vi "Dashboard Main.vi"() -> ()   [LabVIEW 2015]
uses:
  <vilib>/Rock Robotics/Network Tables/NT Read Boolean.vi
  <vilib>/Utility/config.llb/Write Key (String).vi
  <vilib>/Utility/config.llb/Write Key (I32).vi
  <vilib>/event_ctls.llb/eventvkey.ctl
  <vilib>/Utility/config.llb/NI_LVConfig.lvlib
  <vilib>/Rock Robotics/WPI/Dashboard/WPI_DashboardLogging Global.vi
  <vilib>/vision/NI_Vision_Development_Module.lvlib
panel:
  in  "LED Robot Mode":T1(ring)
  out "leds 1":string="RGB LED Control                                                                 "
  in  "LEDs OFF":bool caption="Tare PDP Currents:\nSets current currents to zero,\nlike homing a scale."
  in  "Opening Ceremonies Mode":bool caption="Tare PDP Currents:\nSets current currents to zero,\nlike homing a scale."
  out "leds 2":string="LED Mode Override                                                             "
  in  "Override LED Mode":bool caption="Tare PDP Currents:\nSets current currents to zero,\nlike homing a scale."
  out "leds 3":string="Opening ceremonies mode takes precedence over the mode set using override LED mode."
  out "Chart 2":cluster{"Numeric":dbl, "Numeric":dbl}(graph)
  in  "Notifications":bool
  in  "NotificationCluster":cluster{"Notification Log":i32[]}
  out "notification":string
  out "Robot Mode":T2(ring)
  out "Process?":bool
  in  "Listbox":i32(listbox)
  out "Progress":T3 {"Test Progress" scale=0.0..100.0}
  in  "Motor":cluster{"Value":dbl, "Enable":bool} {"Value" scale=-1.0..1.0 scale format="%#_3g"}
  in  "Test Slider":dbl(slide) scale=0.0..100.0 scale format="%#_3g"
  in  "On/Off":bool caption="Solenoid"
  in  "Test Name":u16(ring) items=["Select the test to run..."]
  in  "Rev/Fwd":cluster{"Forward":bool, "Reverse":bool}
  in  "Test Ring":u16(ring) items=["Monochrome", "Color"]
  in  "Test Tree":string(tree)
  in  "DB/String 9":string
  in  "DB/String 8":string
  in  "DB/String 7":string
  in  "DB/String 6":string
  in  "DB/String 5":string
  in  "DB/String 4":string
  in  "DB/String 3":string
  in  "DB/String 2":string
  in  "DB/String 1":string
  in  "DB/String 0":string
  in  "DB/Slider 0":dbl(slide) scale=0.0..5.0
  in  "DB/Slider 1":dbl(slide) scale=0.0..5.0
  in  "DB/Slider 2":dbl(slide) scale=0.0..5.0
  in  "DB/Slider 3":dbl(slide) scale=0.0..5.0
  out "DB/LED 3":bool
  out "DB/LED 2":bool
  out "DB/LED 1":bool
  out "DB/LED 0":bool
  in  "DB/Button 3":bool
  in  "DB/Button 2":bool
  in  "DB/Button 1":bool
  in  "DB/Button 0":bool caption="New Name"
  in  "TCP":refnum<k5>
  in  "Rec Mode":enum32{"Stop", "Record", "Playback"}(radio)
  out "Camera IP":string
  in  "Dashboard Tab":T4(tab)
  out "Shooter Camera Active":bool
  out "Intake Camera Active":bool
  out "Camera In Targeting Mode":bool
  out "Intake Ball Sensor":bool
  in  "Camera Selector":bool=TRUE
  out "Robot Mode 2":T2(ring)=enum."Disconnected"
  in  "Camera Settings":T5={"Frame Rate"=30, "Compression"=30, "Size"=1} {"Size" items=["640x480", "320x240", "160x120"]; "Frame Rate" scale=1.0..30.0}
  out "Image Message":string="Timeout in Camera Communications"
  out "Camera Image":T6(plugin-control)
  in  "DB Camera Config":bool
  out "fps":dbl format="%#.1g"
  out "Mbps 2":bool
  out "FMS Connection":bool
  out "Dashboard Connection":bool
  out "Robot Connection":bool
  in  "Vision":u16(ring)=2 items=["Camera Off", "USB Camera SW", "USB Camera HW", "IP Camera"]
  out "Mbps":i32 format="%.0f mb/s"
  out "Arm Actuator \nLimit Switches":cluster{"Back":bool, "Forward":bool}
  out "Chart":cluster{"Distance":dbl, "Distance":dbl}(graph)
  out "Gyro":dbl(knob) scale=0.0..360.0 scale format="%#_g°"
  out "Angle":dbl format="%#_g°"
  out "Angular Rate (°/s)":dbl
  in  "Right":bool
  in  "Left":bool
  out "Left Drive":cluster{"Distance":dbl, "Rate":dbl} {"Distance" format="%#_g in"}
  out "MotorSliders L":cluster{"MotorSlide4 2":dbl} {"MotorSlide4 2" scale=0.0..14.0 scale format="%#_2e"}
  out "MotorChart L":cluster{"Battery V":dbl}(graph)
  out "Right Drive":cluster{"Distance":dbl, "Rate":dbl} {"Distance" format="%#_g in"}
  out "Robot IP":string
  out "Camera IP":string
  out "Shooter Rate":dbl format="%#_g rpm"
  out "Arm Actuator Rate":dbl
  out "Arm Actuator Distance":dbl
  out "Targets":T6(plugin-control)
  out "Image":T6(plugin-control)
  in  "Hue Range":cluster{"Lower value":i32, "Upper value":i32}={"Lower value"=80, "Upper value"=120}
  in  "Sat Range":cluster{"Lower value":i32, "Upper value":i32}={"Lower value"=52, "Upper value"=255}
  in  "Luma Range":cluster{"Lower value":i32, "Upper value":i32}={"Lower value"=40, "Upper value"=255}
  out "safety info":string="See Error Log page for more information."
  out "Drive Train":T7
  out "Arm Actuator":T8
  out "Ramp Belts":T9
  out "Shooter":T10
  in  "Error Log":i32(listbox)=-1
  out "CPU Utilization":T11 {"CPU % ISR" format="%#_g%"; "CPU % Time Crit" format="%#_g%"; "CPU % Timed Str" format="%#_g%"; "CPU % High" format="%#_g%"; "CPU % Above" format="%#_g%"; "CPU % Normal" format="%#_g%"; "CPU % Low" format="%#_g%"}
  out "RAM Usage":u32(slide) max=0 scale=-1.0..242810880.0
  out "CPU %":sgl(slide) scale=0.0..100.0
  out "CAN":T12 {"% Bus Utilization" format="%#_g%"}
  out "CAN BUS %":sgl(slide) scale=0.0..100.0
  out "Storage":T13
  out "Current":dbl format="%#_gA"
  out "Temperature":dbl format="%#_g°F"
  out "roboRIO":T14 {"roboRIO V&I"."roboRIO input voltage" format="%#_gV"; "roboRIO V&I"."roboRIO input current" format="%#_gA"}
  out "Rail Voltages":T15 {"6 volt rail"."6 volt rail voltage" format="%#_gV"; "6 volt rail"."6 volt rail current" format="%#_gA"; "5 volt rail"."5 volt rail voltage" format="%#_gV"; "5 volt rail"."5 volt rail current" format="%#_gA"; "3.3 volt rail"."3.3 volt rail voltage" format="%#_gV"; "3.3 volt rail"."3.3 volt rail current" format="%#_gA"}
  out "All Currents (A)":dbl[](array[numeric])
  out "Voltage":dbl format="%#_gV"
  out "PDP Energy":cluster{"Energy":dbl, "Power":dbl} {"Energy" format="%#_gJ"; "Power" format="%#_gW"}
  out "Control Bits":T16
  out "Status Bits":T17
  out "Team Station":u8(ring) items=["Red 1", "Red 2", "Red 3", "Blue 1", "Blue 2", "Blue 3"]
  out "Countdown":sgl
  out "Match Replay":u8
  out "Match Number":u16
  out "Match Type":u8
  out "Event Name":string
  out "Code Trace":T18
  out "Code?":enum16{"unknown", "noCode", "code"}(ring)
  out "Controller Type":enum16{"unknown", "cRIO", "roboRio"}(ring)
  out "Tree":string(tree)
  in  "refresh":bool
  out "Keys":string[](array[string])
  in  "Values":string[](array[string])
  in  "update":bool
  in  "Enable Compressor":bool
  in  "What should the robot do?":T19(ring)
  in  "What defense is in front of the robot?":T20(ring)
  in  "Clear Log":bool caption="Clear Log: This clears the notification\nlog."
  in  "Bottom Right":bool caption="Bottom Right: Moves the notification\nbar to the  bottom right of the screen."
  in  "Bottom Left":bool caption="Bottom Left: Moves the notification\nbar to the bottom left of the screen."
  in  "Top Right":bool caption="Top Right: Moves the notification\nbar to the top right of the screen."
  in  "Top Left":bool caption="Top Left: Moves the notification\nbar to the top left of the screen."
  out "Notifications":bool
  in  "Enable Notifications":bool=TRUE caption="Enable Notifications: Enable the\ndisplaying of important power\nwarnings in a notification pop-up."
  out "hover hint":string="hover over controls for help"
  out "About Selected Auto Mode":string
  in  "Reset Error Log":bool caption="Reset Error Log:\nThis clears all the entries in the error \nlog on the error log tab."
  in  "Clear PDP Sticky Faults":bool caption="Clear PDP Sticky Faults:\nThis resets the faults on the PDP and \nthe associated LEDs. These faults do \nnot clear with a robot reboot."
  in  "Reset PDP Energy":bool caption="Reset PDP Energy:\nResets the PDP energy statistics,\nspecifically the energy (J) and the\npower (W)."
  in  "Dismiss Notification":bool caption="Dismiss Notification: Clears the\ncurrent notification."
  in  "Which defense position is the robot in front of?":enum16{"1", "2", "3", "4", "5", "Spy Box"}(ring)=enum."2"
  out "Dashboard Revision":string
  out "What's connected?":string
  in  "Channel":T21(ring)
  out "Code Revision":string
  out "Time":string
  out "Boolean":bool
  # "1124"
  # "Connections & Robot Status"
  # "Robot Name Goes Here     换"
  # "Don't forget to configure autonomous!"
  # "««       Build Season Alpha Build         »»"
  # "Intake Camera"
  # "Shooter Camera"
  # "General"
  # "Arm Actuator"
  # "Shooter Wheels"
  # "Battery"
  # "Battery"
  # "Default\nValues"
  # "80\n\n\n120"
  # "52\n\n\n255"
  # "40\n\n\n255"
  # "Robot Metrics"
  # "See the below driver station for\ngraphs of CPU%"
  # "PDP Data"
  # "General"
  # "Event & Match Info"
  # "This controls the roboRIO's local config file and \npersists after reboots. \n\nThis data is roboRIO\nspecific and only affects the currently connected\nroboRIO. \n\nOnly edit these if you know what you are doing.\nPlease."
  # "Power Commands"
  # "Notifications"
  # "Power Distribution Panel"
  # "Only do this when\nthe compressor\nis connected!"
  # "Autonomous Configuration"
  # "Error Log Controls"
  # "Screen Location"
  # "Help"
  # "Power Distribution Panel Channels"
  # "ÜberBots Team 1124"
  # "CAN Line for Talon SRX in Parentheses if Applicable"
  # "ÜberDashboard 2015"
  # "Power Distribution Panel"
  # "CH 0"
  # "CH 3"
  # "CH 2"
  # "CH 1"
  # "CH 6"
  # "CH 7"
  # "CH 5"
  # "CH 4"
  # "CH 12"
  # "CH 13"
  # "CH 14"
  # "CH 15"
  # "CH 8"
  # "CH 9"
  # "CH 10"
  # "CH 11"
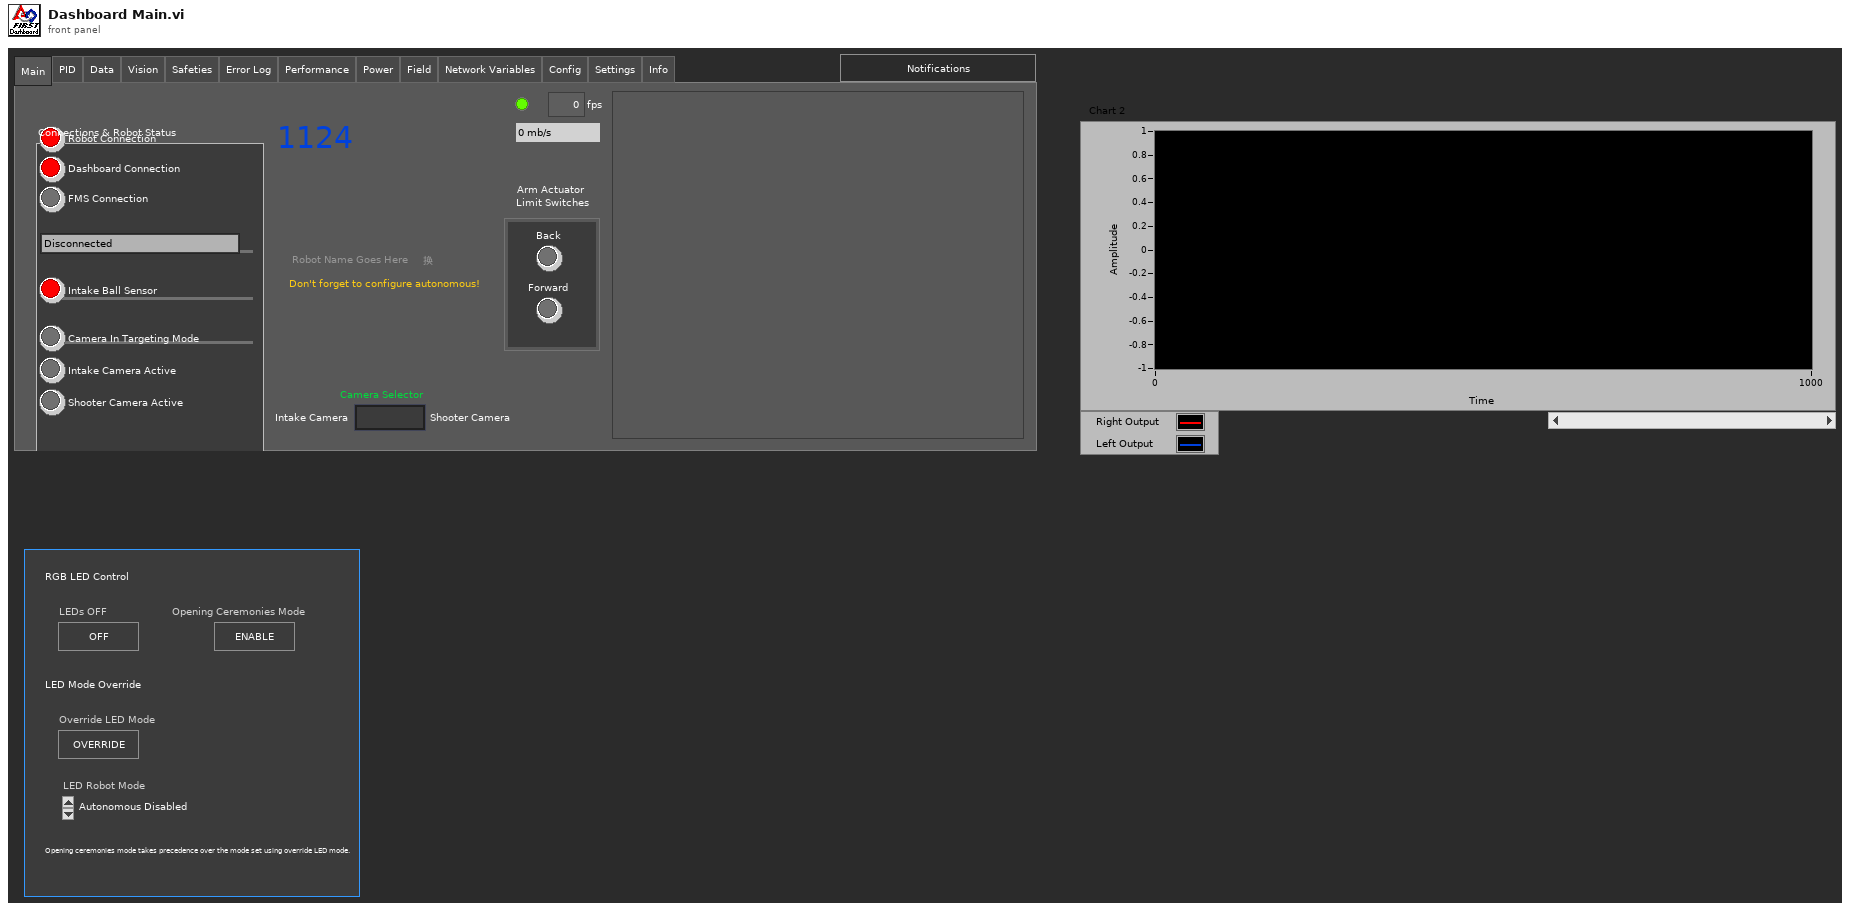
[diagram p1: front panel]
types:
  T1 = enum16{"Autonomous Disabled", "Autonomous Enabled", "Teleop Disabled", "Teleop Enabled", "Disconnected", "Finish", "Test Disabled", "Test Enabled", "Emergency Stopped"}
  T2 = enum8{"Tele-Op Disabled", "Tele-Op Enabled", "Auto Disabled", "Auto Enabled", "Test Disabled", "Test Enabled", "Disconnected", "No Code", "E-Stop"}
  T3 = cluster{"Test Progress":u8, "Test Progress Text":string}
  T4 = enum32{"Main", "PID", "Data", "Vision", "Safeties", "Error Log", "Performance", "Power", "Field", "Network Variables", "Config", "Settings", "Info"}
  T5 = cluster{"Frame Rate":i32, "Compression":i32, "Size":u16}
  T6 = typedef "IMAQ Image.ctl" = refnum<image>
  T7 = cluster{"Left Disconnected [inf]":bool, "Left Disconnected [zero]":bool, "Right Disconnected [inf]":bool, "Right Disconnected [zero]":bool}
  T8 = cluster{"Arm Actuator Limit Switch":bool, "Arm Actuator Encoder Limit":bool, "Arm Actuator Disconnected [inf]":bool, "Arm Actuator Disconnected [zero]":bool}
  T9 = cluster{"Ramp Belts Disconnected [inf]":bool, "Ramp Belts Disconnected [zero]":bool}
  T10 = cluster{"Shooter Disconnected [inf]":bool, "Shooter Disconnected [zero]":bool}
  T11 = cluster{"CPU % ISR":sgl, "CPU % Time Crit":sgl, "CPU % Timed Str":sgl, "CPU % High":sgl, "CPU % Above":sgl, "CPU % Normal":sgl, "CPU % Low":sgl}
  T12 = cluster{"% Bus Utilization":sgl, "Bus Off Cnt":u32, "TX_FIFO Full Cnt":u32, "Receive Error Cnt":u8, "Transmit Error Cnt":u8}
  T13 = cluster{"Disk Free":u64, "RAM Block":u32, "RAM free":u32}
  T14 = cluster{"roboRIO V&I":cluster{"roboRIO input voltage":dbl, "roboRIO input current":dbl}, "roboRIO Enables":cluster{"3.3V Enabled":bool, "5 V Enabled":bool, "6 V Enabled":bool}}
  T15 = cluster{"6 volt rail":cluster{"6 volt rail voltage":dbl, "6 volt rail current":dbl, "6 volt rail fault count":dbl}, "5 volt rail":cluster{"5 volt rail voltage":dbl, "5 volt rail current":dbl, "5 volt rail fault count":dbl}, "3.3 volt rail":cluster{"3.3 volt rail voltage":dbl, "3.3 volt rail current":dbl, "3.3 volt rail fault count":dbl}}
  T16 = cluster{"Test Mode":bool, "Autonomous":bool, "Enabled":bool, "FMS Present":bool, bool, bool, bool, "E-Stop":bool}
  T17 = cluster{"Test Mode":bool, "Autonomous":bool, "Enabled":bool, "Code Start":bool, "Brownout":bool, "Reserved 2":bool, "Reserved 3":bool, "E-Stop":bool}
  T18 = cluster{"Disabled":bool, "TeleOp":bool, "Auto":bool, "Test":bool}
  T19 = enum16{"Nothing at all", "Get to Defense", "Cross Defense", "Score High Goal", "Score Low Goal"}
  T20 = enum16{"Moat", "Ramparts", "Rock Wall", "Rough Terrain", "Something Else"}
  T21 = enum16{"0", "1", "2", "3", "4", "5", "6", "7", "8", "9", "10", "11", "12", "13", "14", "15"}
  T22 = typedef "Image Type" = u32
  T23 = enum32{"Drive", "Basic", "Custom", "Test", "Checklist", "Variables"}
  T24 = cluster{"Camera Image":refnum<vi>, "Dashboard Tab":refnum<vi>, "Boolean":refnum<vi>, "Vision":refnum<vi>, "Rec Mode":refnum<vi>, "Test Slider":refnum<vi>, "On/Off ":refnum<vi>, "Test Ring":refnum<vi>, "Rev/Fwd":refnum<vi>, "Test Name":refnum<vi>, "Motor":refnum<vi>, "Progress":refnum<vi>, "CheckList":refnum<vi>, "Tree":refnum<vi>, "Test Tree":refnum<vi>}
  T25 = cluster{"Error Strings":string, "Disable Counts":cluster{u16, u16}, "Rail Faults":cluster{u16, u16, u16}, "Robot IP":string, "DB Mode":u8, "Event Info":cluster{"Name":string, "Type":u8, "Number":u16, "Replay":u8}, "Camera Addr":string}
  T26 = cluster{"Storage":cluster{"Disk Free":u64, "RAM Block":u32, "RAM free":u32}, "CPU Utilization":cluster{"CPU % ISR":sgl, "CPU % Time Crit":sgl, "CPU % Timed Str":sgl, "CPU % High":sgl, "CPU % Above":sgl, "CPU % Normal":sgl, "CPU % Low":sgl}, "CAN":cluster{"% Bus Utilization":sgl, "Bus Off Cnt":u32, "TX_FIFO Full Cnt":u32, "Receive Error Cnt":u8, "Transmit Error Cnt":u8}, "HID":cluster{"HID Outputs":u32, "Rumble Low":u16, "Rumble High":u16}[]}
  T27 = cluster{"Status bits":cluster{"Test Mode":bool, "Autonomous":bool, "Enabled":bool, "Code Start":bool, "Brownout":bool, "Reserved 2":bool, "Reserved 3":bool, "E-Stop":bool}, "Code Trace":cluster{"Disabled":bool, "TeleOp":bool, "Auto":bool, "Test":bool}, "Controller Type":enum16{"unknown", "cRIO", "roboRio"}, "Code?":enum16{"unknown", "noCode", "code"}, "Battery V":dbl}
  T28 = cluster{"Control Bits":cluster{"TestMode":bool, "Autonomous":bool, "Enabled":bool, "FMS Present":bool, bool, bool, bool, "E-Stop":bool}, "Team Station ":u8, "Countdown":sgl, "Joystick Values":cluster{"Axes":dbl[], "Buttons":bool[], "POVs":i16[]}[]}
  T29 = cluster{"TestMode":bool, "Autonomous":bool, "Enabled":bool, "FMS Present":bool, bool, bool, bool, "E-Stop":bool}
  T30 = cluster{"Axes":dbl[], "Buttons":bool[], "POVs":i16[]}[]
  T31 = cluster{"Axes":dbl[], "Buttons":bool[], "POVs":i16[]}
  T32 = cluster{"roboRIO V&I":cluster{"roboRIO input voltage (V)":dbl, "roboRIO input current (A)":dbl}, "roboRIO Enabled":cluster{"3.3V Enabled":bool, "5 V Enabled":bool, "6 V Enabled":bool}}
  T33 = cluster{"6 volt rail":cluster{"6 volt rail voltage (V)":dbl, "6 volt rail current (A)":dbl, "6 volt fault count":dbl}, "5 volt rail":cluster{"5 volt rail voltage (V)":dbl, "5 volt rail current (A)":dbl, "5 volt fault count":dbl}, "3.3 volt rail":cluster{"3.3 volt rail voltage (V)":dbl, "3.3 volt rail current (A)":dbl, "3.3 volt fault count":dbl}}
  T34 = cluster{"all currents (A)":dbl[], "PDP Energy":cluster{"Energy (J)":dbl, "Power (W)":dbl}, "voltage (V)":dbl, "temperature (F)":dbl, "current (A)":dbl}
  T35 = cluster{"Safety Data Prev Iteration":bool[][], "Item Names":string[][]}
  T36 = cluster{"Operation":enum16{"Update", "Clear"}, "Color Box":u32}[]
  T37 = typedef "eventvkey.ctl" = enum16{"ASCII", "Enter", "Return", "Shift", "Ctrl", "Alt", "Cmd", "Opt", "Caps", "NumLock", "Clear", "Break", "Up", "Down", "Left", "Right", "Insert", "Delete", "Home", "End", "PageUp", "PageDown", "Escape", "Help", "Pause", "ScrollLock", "F1", "F2", "F3", "F4", "F5", "F6", "F7", "F8", "F9", "F10", "F11", "F12", "F13", "F14", "F15", "F16", "F17", "F18", "F19", "F20", "F21", "F22", "F23", "F24", "Play", "VolumeUp", "VolumeDown", "Mute", "Two Byte Char"}
  T38 = cluster{"Image Size":bool, "Image Type":bool, "Pixel Value":bool, "ROI Information":bool, "Zoom Factor":bool}
  T39 = enum8{"Enabled", "Disabled", "Disabled and Grayed Out"}
  T40 = typedef "NI_LVConfig.lvlib/Config Data RefNum.ctl" = refnum<k1>
  T41 = cluster{"Operation":enum16{"Update", "Clear"}, "Color Box":u32}
  T42 = typedef "LVPositionTypeDef.ctl" = cluster{"Left":i32, "Top":i32}
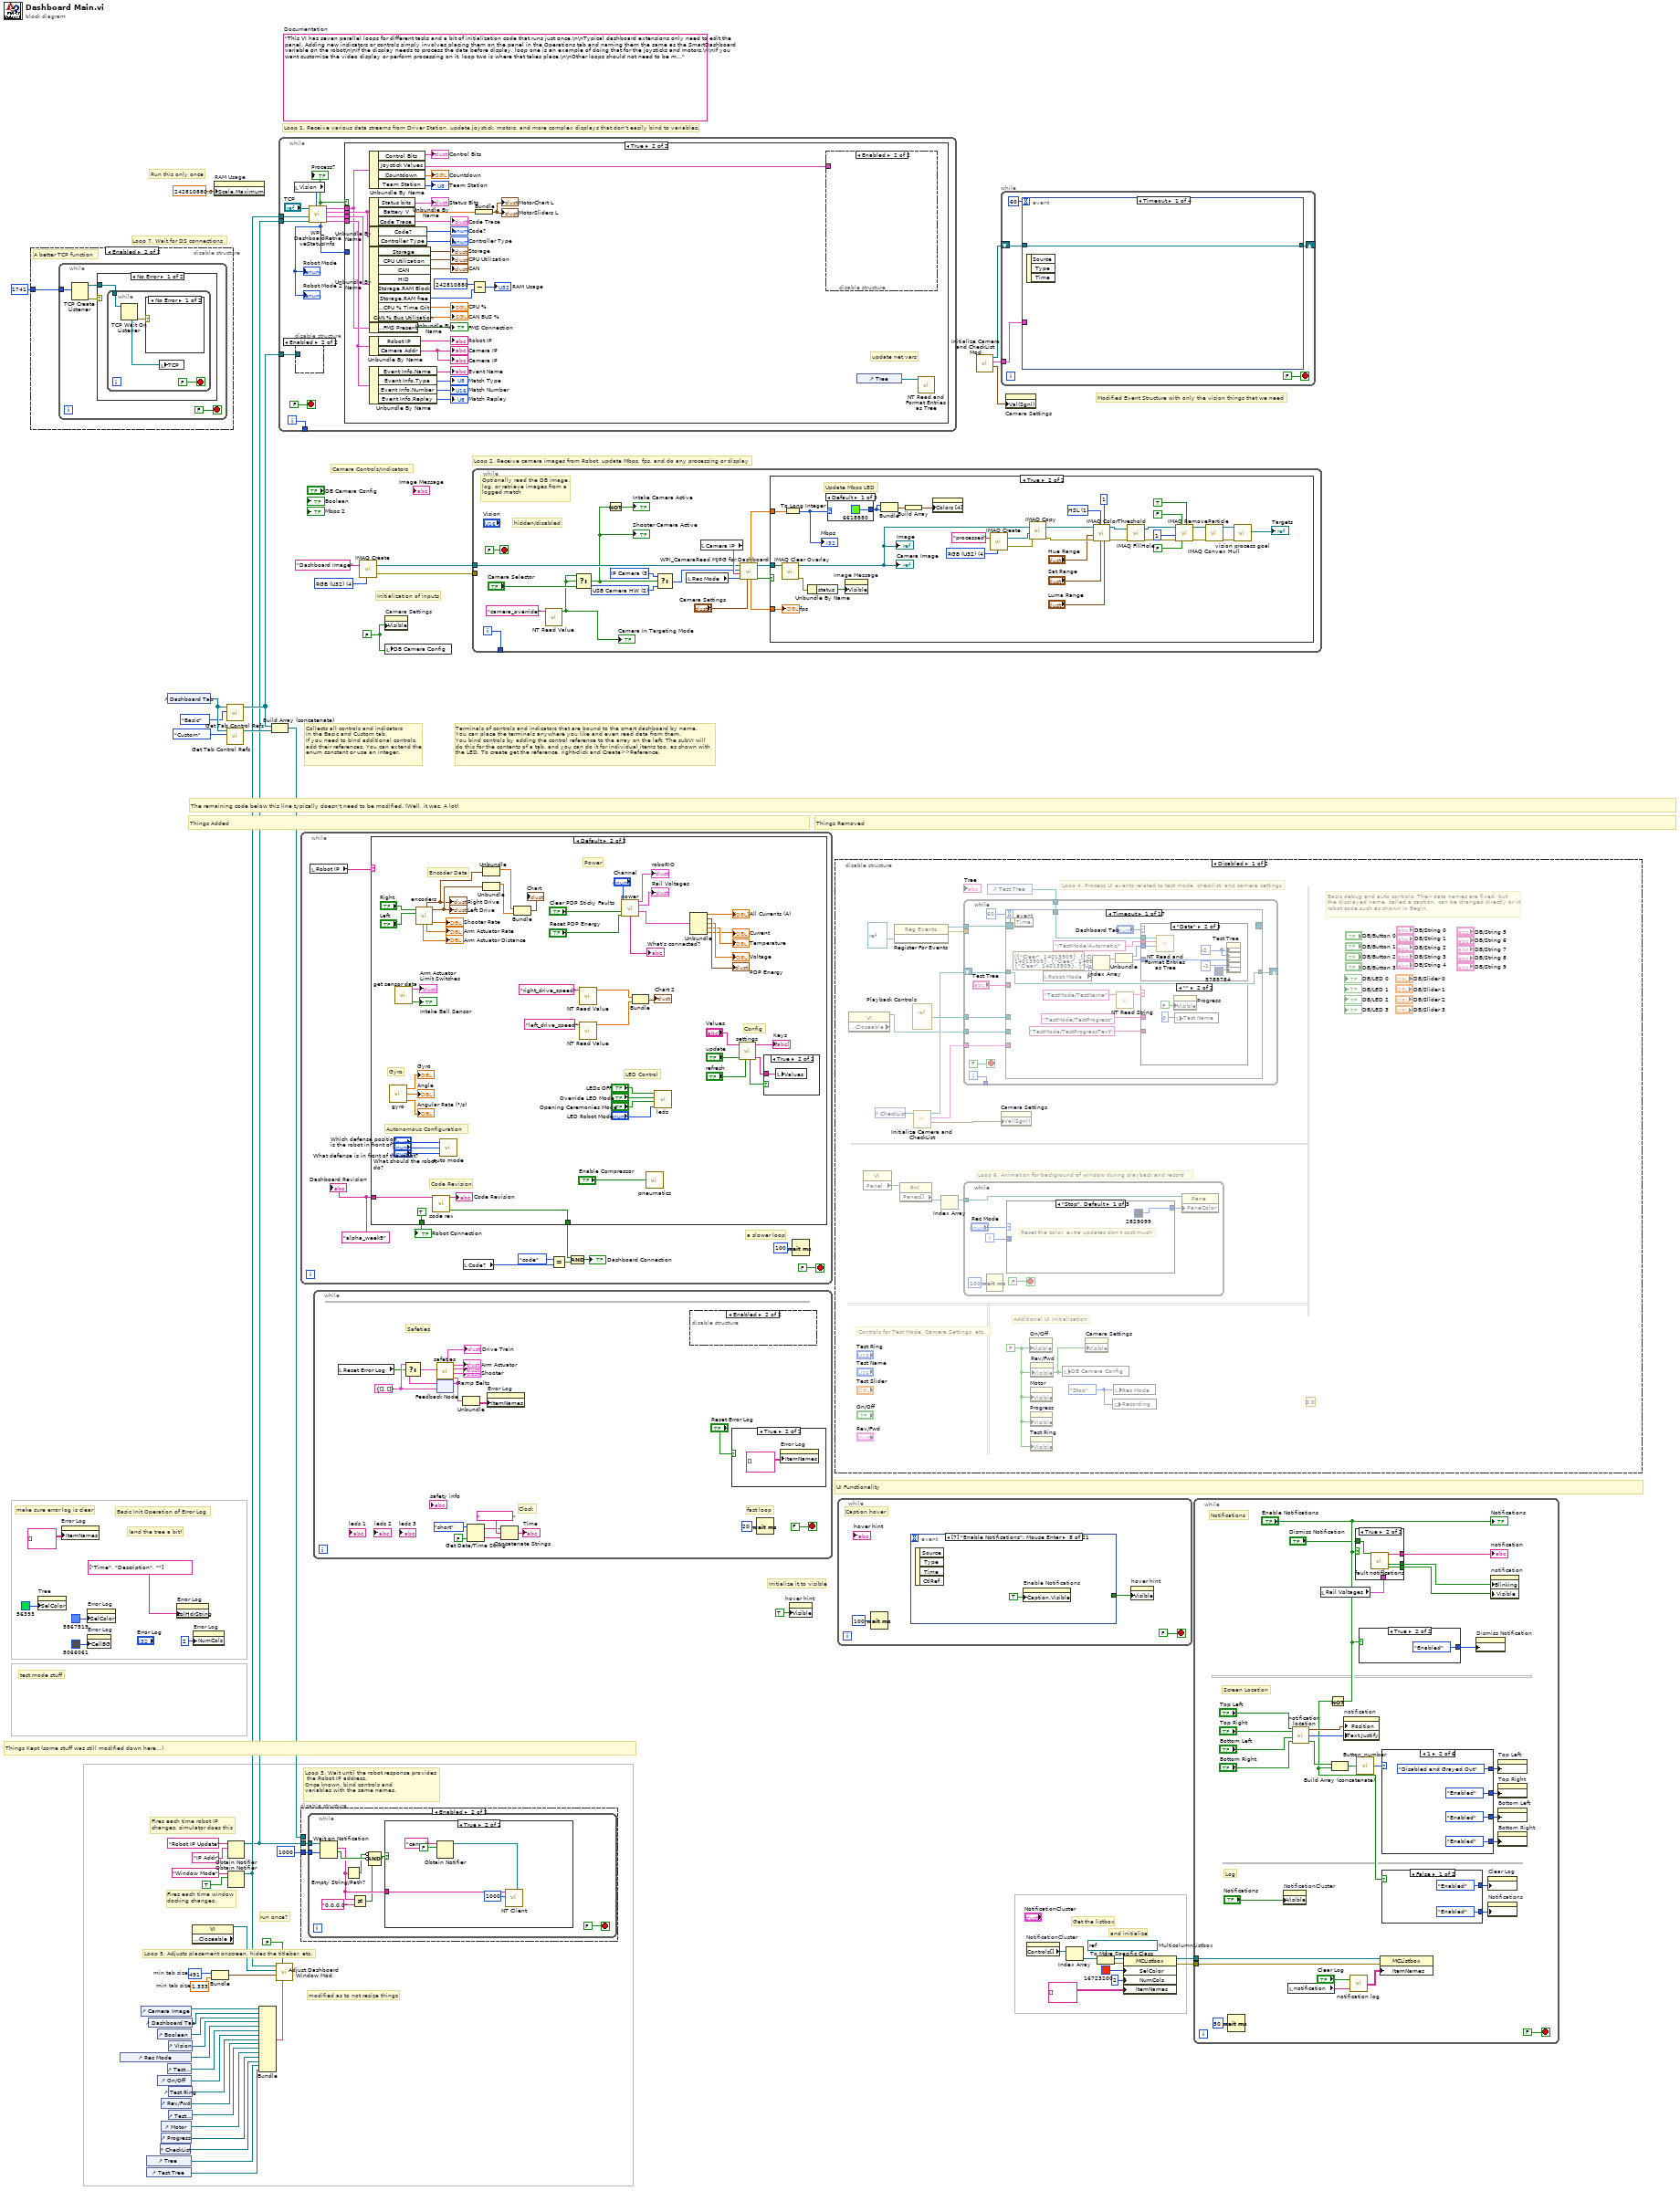
[diagram p0: block diagram]
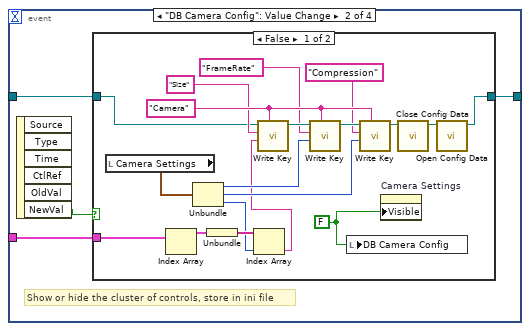
[diagram p2: hidden frame]
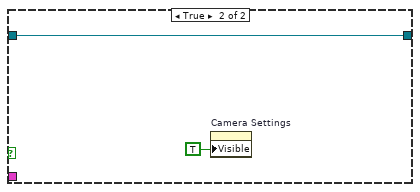
[diagram p3: hidden frame]
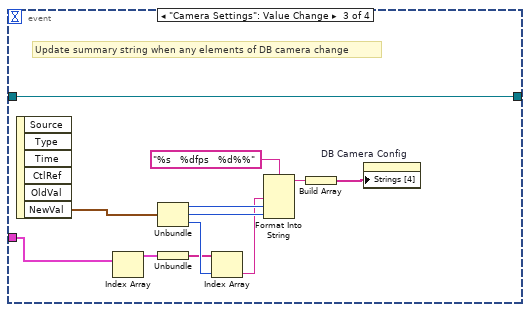
[diagram p4: hidden frame]
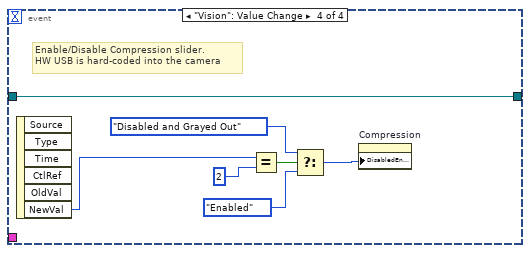
[diagram p5: hidden frame]
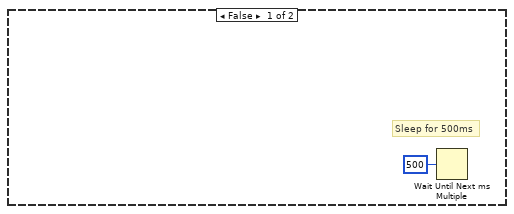
[diagram p6: hidden frame]
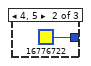
[diagram p7: hidden frame]
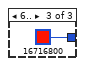
[diagram p8: hidden frame]
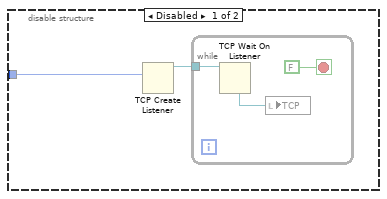
[diagram p9: hidden frame]
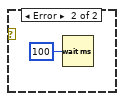
[diagram p10: hidden frame]
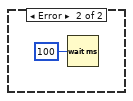
[diagram p11: hidden frame]
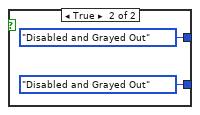
[diagram p12: hidden frame]
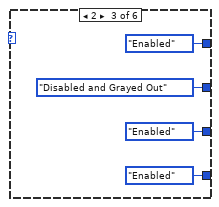
[diagram p14: hidden frame]
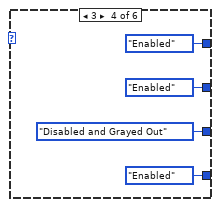
[diagram p15: hidden frame]
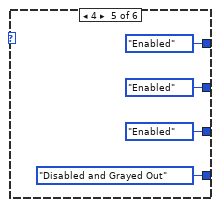
[diagram p16: hidden frame]
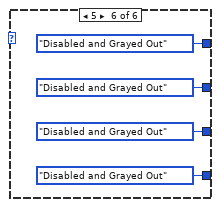
[diagram p17: hidden frame]
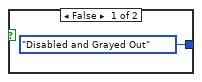
[diagram p18: hidden frame]
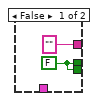
[diagram p19: hidden frame]
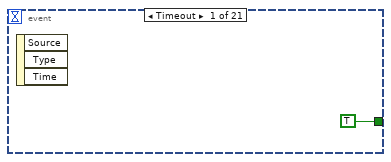
[diagram p20: hidden frame]
diagram:
  w1 = FALSE ("DB Camera Config")
  w7 = T22 4 items=["Grayscale (U8)", "Grayscale (I16)", "Grayscale (SGL)", "Complex (CSG)", "RGB (U32)", "HSL (U32)", "RGB (U64)"] ("Image Type")
  w16 = refnum<vi> refnum  # MulticolumnListbox
  w50 = 491  # min tab size
  w49 = 1.333  # min tab size
  (unwired) "This VI has seven parallel loops for different tasks and a bit of initialization code that runs just once.\n\nTypical dashboard extensions only need to edit the panel. Adding new indicators or controls simply involves placing them on the panel in the Operations tab and naming them the same as the SmartDashboard variable on the robot\n\nIf the display needs to process the data before display, loop one is an example of doing that for the joysticks and motors.\n\nIf you want customize the video display or perform processing on it, loop two is where that takes place.\n\nOther loops should not need to be modified. They are pretty standard, and document the task they perform."  # Documentation
  # "Camera Controls/Indicators"
  # "Modified Event Structure with only the vision things that we need"
  # "Initialization of inputs"
  # "Loop 2. Receive camera images from Robot, update Mbps, fps, and do any processing or display"
  # "Loop 7. Wait for DS connections"
  # "Run this only once"
  # "test mode stuff"
  # "and initialize"
  # "Get the listbox"
  # "Initialize it to visible"
  # "UI Functionality"
  # "(and the tree a bit)"
  # "run once?"
  # "make sure error log is clear"
  # "Basic Init Operation of Error Log"
  # "modified as to not resize things"
  # "Things Kept (some stuff was still modified down here...)"
  # "Things Added"
  # "Things Removed"
  # "Fires each time robot IP\nchanges, simulator does this"
  # "Fires each time window\ndocking changes."
  # "Collects all controls and indicators\nin the Basic and Custom tab.\nIf you need to bind additional controls,\nadd their references. You can extend the\nenum constant or use an integer."
  # "The remaining code below this line typically doesn't need to be modified. (Well, it was. A lot)"
  # "Terminals of controls and indicators that are bound to the smart dashboard by name.\nYou can place the terminals anywhere you like and even read data from them.\nYou bind controls by adding the control reference to the array on the left. The subVI will\ndo this for the contents of a tab, and you can do it for individual items too, as shown with\nthe LED. To create get the reference, right-click and Create>>Reference."
  # "Loop 3. Wait until the robot response provides\n the Robot IP address.\nOnce known, bind controls and\nvariables with the same names."
  # "Loop 5. Adjusts placement onscreen, hides the titlebar, etc."
  # "Loop 1. Receive various data streams from Driver Station, update joystick, motors, and more complex displays that don't easily bind to variables."
  n1 = disable-structure shown="Enabled" {
    disable-tunnel: u16 1741 ("timeout ms (25000)") -> [w63 w67]
    frame Disabled {
      n2 = TCP Create Listener(10:w63) -> (3:w62:refnum<k5>)  [unwired: 4 in, 2 out]
      n3 = while {
        tunnel: w62 -> [w66]
        stop <- FALSE stop-if-true
        n4 = TCP Wait On Listener(11:w66) -> (4:w65:refnum<k5>)  [unwired: 3 in, 4 out]
        n5 = local write "TCP"(w65) -> ()
      }
    }
    frame Enabled {
      # "A better TCP function"
      n6 = while {
        tunnel: w67 -> [w70]
        stop <- FALSE stop-if-true
        n7 = TCP Create Listener(10:w70) -> (0:w69:errorcluster, 3:w68:refnum<k5>)  [unwired: 4 in, 1 out]
        n8 = case shown="No Error" w69 {
          tunnel: w68 -> [w72 _]
          frame No Error {
            n9 = while {
              tunnel: w72 -> [w74]
              stop <- FALSE stop-if-true
              n10 = TCP Wait On Listener(11:w74) -> (0:w73:errorcluster, 4:w75:refnum<k5>)  [unwired: 3 in, 3 out]
              n11 = case shown="No Error" w73 {
                frame No Error {
                }
                frame Error {
                  n12 = Wait (ms)(milliseconds to wait=u32 100) -> ()  [unwired: 1 out]
                }
              }
              n13 = local write "TCP"(w75) -> ()
            }
          }
          frame Error {
            n14 = Wait (ms)(milliseconds to wait=u32 100) -> ()  [unwired: 1 out]
          }
        }
      }
    }
  }
  n15 = property on="Tree" class="Tree (strict)"("SelColor"=u32 56393 ("Round Color Box")) -> ()  [unwired: 2 in, 2 out]
  n16 = property on="Error Log" class="MCListbox (strict)"("ItemNames"=string[][] [] ("Item Names")) -> ()  [unwired: 2 in, 2 out]
  n17 = property on="Error Log" class="MCListbox (strict)"("SelColor"=u32 5867519 ("Round Color Box")) -> ()  [unwired: 2 in, 2 out]
  n18 = property on="Error Log" class="MCListbox (strict)"("CellBG"=u32 5066061 ("Round Color Box")) -> ()  [unwired: 2 in, 2 out]
  n19 = control-ref of="Rec Mode"() -> (w41:refnum<vi>)
  n20 = control-ref of="Camera Image"() -> (w53:refnum<vi>)
  n21 = control-ref of="Tree"() -> (w45:refnum<vi>)
  n22 = control-ref of="Test Tree"() -> (w44:refnum<vi>)
  n23 = control-ref of="Dashboard Tab"() -> (w52:refnum<vi>)
  n24 = control-ref of="Boolean"() -> (w48:refnum<vi>)
  n25 = control-ref of="On/Off"() -> (w39:refnum<vi>)
  n26 = control-ref of="CheckList"() -> (w34:refnum<vi>)
  n27 = control-ref of="Rev/Fwd"() -> (w37:refnum<vi>)
  n28 = control-ref of="Motor"() -> (w42:refnum<vi>)
  n29 = control-ref of="Progress"() -> (w36:refnum<vi>)
  n30 = control-ref of="Dashboard Tab"() -> (w56:refnum<vi>)
  n31 = control-ref of="Test Slider"() -> (w40:refnum<vi>)
  n32 = control-ref of="Vision"() -> (w51:refnum<vi>)
  n33 = control-ref of="Test Ring"() -> (w38:refnum<vi>)
  n34 = control-ref of="Test Name"() -> (w43:refnum<vi>)
  n35 = property on="Error Log" class="MCListbox (strict)"("ColHdrString"=string[] ["Time", "Description", ""] ("Column Header Strings[]")) -> ()  [unwired: 2 in, 2 out]
  n36 = property class="VI" props=["Front Panel.Closeable"]() -> (reference out=w31:refnum<vi>)  [unwired: 2 in, 2 out]
  n37 = property on="Error Log" class="MCListbox (strict)"("NumCols"=u32 2 ("Number of Columns")) -> ()  [unwired: 2 in, 2 out]
  n38 = Bundle("min tab size"=w50, "min tab size"=w49) -> (w32:cluster{"min tab size":i32, "min tab size":dbl})  [unwired: 1 in]
  n39 = property on="RAM Usage" class="Slide (strict)"("Scale.Maximum"=242810880.0) -> ()  [unwired: 2 in, 2 out]
  n40 = call <vilib>:"Get Tab Control Refs.vi"("Page Index"=T23."Basic" ("Dashboard Tab"), "TabControl in"=w56) -> ("ControlsOnPage"=w35:refnum<vi>[])  [unwired: 9 in]
  n41 = call <vilib>:"Get Tab Control Refs.vi"("Page Index"=T23."Custom" ("Dashboard Tab"), "TabControl in"=w56) -> ("ControlsOnPage"=w55:refnum<vi>[])  [unwired: 9 in]
  n42 = Obtain Notifier(name (unnamed)="Robot IP Update", notification data type="IP Addr" ("name (unnamed)")) -> (notifier out=w29:refnum<notifier>)  [unwired: 2 in, 2 out]
  n43 = Obtain Notifier(name (unnamed)="Window Mode", notification data type=TRUE) -> (notifier out=w30:refnum<notifier>)  [unwired: 2 in, 2 out]
  n44 = Bundle("Camera Image"=w53, "Dashboard Tab"=w52, "Boolean"=w48, "Vision"=w51, "Rec Mode"=w41, "Test Slider"=w40, "On/Off"=w39, "Test Ring"=w38, "Rev/Fwd"=w37, "Test Name"=w43, "Motor"=w42, "Progress"=w36, "CheckList"=w34, "Tree"=w45, "Test Tree"=w44) -> (w33:T24)  [unwired: 1 in]
  n45 = Build Array (concatenate)(w35, w55) -> (w54:refnum<vi>[])
  n46 = call "Adjust Dashboard Window Mod.vi"("Sizing Refnums"=w33, "Stop?"=FALSE, "Size Constraints"=w32, "VI"=w31, "Notifier in"=w30) -> ()  [unwired: 7 in]
  n47 = while {
    tunnel: [w91] -> _
    tunnel: w29 -> [w85]
    tunnel: w35 -> [w84]
    tunnel: w30 -> [w81]
    i -> [w91]
    stop <- FALSE stop-if-true
    n48 = local read "Vision"() -> (w83:u16)
    n49 = disable-structure shown="Enabled" {
      disable-tunnel: w84 -> [w92 _]
      frame Disabled {
        n50 = call <vilib>:"WPI_DashboardUpdateNames.vi"("Controls on Tab"=w92) -> ()  [unwired: 11 in]
      }
      frame Enabled {
      }
    }
    n51 = call <vilib>:"WPI_DashboardRetrieveStatusInfo.vi"("Vision"=w83, "Binding Refnum"=w85, "Window Mode Notifier"=w81, "TCP Cnx"="TCP") -> ("Power and Errors"=w86:T25, "Robot Metrics"=w89:T26, "Status Info"=w90:T27, "Control Info"=w87:T28, "Robot Mode"=w79:T2, "Process?"=w88:bool)  [unwired: 2 in]
    "Process?" <- w88
    "Robot Mode" <- w79
    "Robot Mode 2" <- w79
    n52 = case shown="True" w88 {
      tunnel: w90 -> [_ w104]
      tunnel: w89 -> [_ w122]
      tunnel: w87 -> [_ w101]
      tunnel: w86 -> [_ w115]
      tunnel: w79 -> [_ _]
      frame False {
      }
      frame True {
        # "update net vars"
        n53 = Unbundle By Name(w101) -> ("Control Bits"=→"Control Bits":T29, "Joystick Values"=w93:T30, "Countdown"=→"Countdown":sgl, "Team Station"=→"Team Station":u8)
        n54 = Unbundle By Name(w104) -> ("Status bits"=→"Status Bits":T17, "Battery V"=w121:dbl, "Code Trace"=→"Code Trace":T18)
        n55 = Unbundle By Name(w104) -> ("Code?"=→"Code?":enum16{"unknown", "noCode", "code"}, "Controller Type"=→"Controller Type":enum16{"unknown", "cRIO", "roboRio"})
        n56 = Unbundle By Name(w122) -> ("Storage"=→"Storage":T13, "CPU Utilization"=→"CPU Utilization":T11, "CAN"=→"CAN":T12, "Storage.RAM free"=w96:u32, "CPU Utilization.CPU % Time Crit"=→"CPU %":sgl, "CAN.% Bus Utilization"=→"CAN BUS %":sgl)  [unwired: 2 out]
        n57 = Unbundle By Name(w101) -> ("Control Bits.FMS Present"=→"FMS Connection":bool)
        n58 = Unbundle By Name(w115) -> ("Robot IP"=→"Robot IP":string, "Camera Addr"=→"Camera IP" →"Camera IP":string)
        n59 = Unbundle By Name(w115) -> ("Event Info.Name"=→"Event Name":string, "Event Info.Type"=→"Match Type":u8, "Event Info.Number"=→"Match Number":u16, "Event Info.Replay"=→"Match Replay":u8)
        n60 = Subtract(x=u32 242810880, y=w96) -> (x-y=→"RAM Usage":u32)
        n61 = Bundle("Battery V"=w121) -> (→"MotorSliders L" →"MotorChart L":cluster{"Battery V":dbl})  [unwired: 1 in]
        n62 = disable-structure shown="Enabled" {
          disable-tunnel: w93 -> [w126 _]
          frame Disabled {
            n63 = Index Array(array=w126) -> (element #1=w125:T31, element #2=w124:T31, element #3=w123:T31)  [unwired: 3 in]
            n64 = call "Prepare Joystick Data for Displays.vi"("Joystick Values"=w124) -> ()  [unwired: 6 in, 5 out]
            n65 = call "Prepare Joystick Data for Displays.vi"("Joystick Values"=w123) -> ()  [unwired: 6 in, 5 out]
            n66 = call "Prepare Joystick Data for Displays.vi"("Joystick Values"=w125) -> ()  [unwired: 6 in, 5 out]
          }
          frame Enabled {
          }
        }
        n67 = control-ref of="Tree"() -> (w105:refnum<vi>)
        n68 = call <vilib>:"NT Read and Format Entries as Tree.vi"("Tree Refnum"=w105) -> ()  [unwired: 9 in, 2 out]
      }
    }
  }
  n69 = disable-structure shown="Enabled" {
    disable-tunnel: u32 1000 ("milliseconds to wait") -> [w129 w146]
    disable-tunnel: w54 -> [w128 _]
    disable-tunnel: w29 -> [w127 w145]
    frame Disabled {
      n70 = while {
        tunnel: w128 -> [w141]
        tunnel: w127 -> [w139]
        tunnel: [w137] -> _
        tunnel: w129 -> [w136]
        i -> [w137]
        stop <- FALSE stop-if-true
        n71 = local read "Rec Mode"() -> (w132:enum32{"Stop", "Record", "Playback"})
        n72 = Wait on Notification(notifier=w139, timeout in ms (-1)=w136) -> (notification=w138:string, timed out?=w134:bool)  [unwired: 2 in, 2 out]
        n73 = Equal?(x=w132, y=u16 2 ("Rec Mode")) -> (x = y?=w133:bool)
        n74 = Compound Arithmetic op=OR(invert w134, w133) -> (w135:bool)
        n75 = case shown="True" w135 {
          tunnel: w141 -> [_ w144]
          tunnel: w138 -> [_ w143]
          tunnel: "Dashboard" -> [_ w142]
          frame False {
          }
          frame True {
            n76 = call <vilib>:"Bind Controls to SmartDashboard.vi"("Client Name"=w142, "Bound Control Refs"=w144, "Server IP Address"=w143) -> ()  [unwired: 9 in]
          }
        }
      }
    }
    frame Enabled {
      n77 = while {
        tunnel: w146 -> [w154]
        tunnel: w145 -> [w153]
        stop <- FALSE stop-if-true
        n78 = Wait on Notification(notifier=w153, timeout in ms (-1)=w154) -> (notification=w149:string, timed out?=w152:bool)  [unwired: 2 in, 2 out]
        n79 = Empty String/Path?(string/path=w149) -> (empty?=w151:bool)
        n80 = Not Equal?(x=w149, y="0.0.0.0") -> (x != y?=w147:bool)
        n81 = Compound Arithmetic op=AND(invert w151, invert w152, w147) -> (w150:bool)
        n82 = case shown="True" w150 {
          tunnel: w149 -> [_ w160]
          frame False {
          }
          frame True {
            n83 = Obtain Notifier(name (unnamed)="cancel", notification data type=FALSE) -> (notifier out=w157:refnum<notifier>)  [unwired: 2 in, 2 out]
            n84 = call <vilib>:"NT Client.vi"("Cancel Ref"=w157, "timeout ms (1000)"=1000, "Server IP Address"=w160) -> ()  [unwired: 9 in]
          }
        }
      }
    }
  }
  n85 = while {
    stop <- FALSE stop-if-true
    w161 = "alpha_week5" ("Dashboard Revision")
    # "a slower loop"
    n86 = local read "Robot IP"() -> (w169:string)
    n87 = case shown="Default" w169 {
      tunnel: [w171 TRUE ("Robot Connection")] -> w168
      tunnel: [w171 w212] -> w163
      tunnel: w161 -> [_ w211]
      frame "", "0.0.0.0" {
        (unwired) dbl[] [] ("motor array")
        w171 = FALSE ("Robot Connection")
      }
      frame Default {
        # "LED Control"
        # "Autonomous Configuration"
        # "Power"
        # "Config"
        # "Code Revision"
        # "Encoder Data"
        # "Gyro"
        n88 = call "gyro.vi"() -> ("Angle"=→"Gyro":dbl, "Full Angle"=→"Angle":dbl, "Angular Rate"=→"Angular Rate (°/s)":dbl)  [unwired: 6 in]
        n89 = call "get sensor data.vi"() -> ("Ramp Belts Light Sensor"=→"Intake Ball Sensor":bool, "Arm Actuator Limit Switches"=→"Arm Actuator \nLimit Switches":cluster{"Boolean":bool, "Boolean":bool})  [unwired: 10 in]
        n90 = call "encoders.vi"("Left"="Left", "Right"="Right") -> ("Shooter Rate"=→"Shooter Rate":dbl, "Left Drive"=w193:cluster{"Distance":dbl, "Rate":dbl}, "Arm Actuator Rate"=→"Arm Actuator Rate":dbl, "Right Drive"=w192:cluster{"Distance":dbl, "Rate":dbl}, "Arm Actuator Distance"=→"Arm Actuator Distance":dbl)  [unwired: 5 in]
        "Right Drive" <- w192
        "Left Drive" <- w193
        n91 = call "code rev.vi"("Dashboard Revision"=w211) -> ("Found Revision"=w212:bool, "Code Revision"=→"Code Revision":string)  [unwired: 9 in]
        n92 = call "auto mode.vi"("What should the robot do?"="What should the robot do?", "What defense is in front of the robot?"="What defense is in front of the robot?", "Which defense position is the robot in front of?"="Which defense position is the robot in front of?") -> ()  [unwired: 1 in]
        n93 = Unbundle(w192) -> ("Distance"=w191:dbl)  [unwired: 1 out]
        n94 = Unbundle(w193) -> ("Distance"=w190:dbl)  [unwired: 1 out]
        n95 = Bundle("Distance"=w191, "Distance"=w190) -> (→"Chart":cluster{"Distance":dbl, "Distance":dbl})  [unwired: 1 in]
        n96 = call-poly <vilib>:"NT Read Value.vi"("Name"="right_drive_speed") -> ("Numeric"=w182:dbl)  [unwired: 9 in, 1 out]
        n97 = call-poly <vilib>:"NT Read Value.vi"("Name"="left_drive_speed") -> ("Numeric"=w181:dbl)  [unwired: 9 in, 1 out]
        n98 = call "power.vi"("Channel"="Channel", "Clear PDP Sticky Faults"="Clear PDP Sticky Faults", "Reset PDP Energy"="Reset PDP Energy") -> ("roboRIO"=→"roboRIO":T32, "Rail Voltages"=→"Rail Voltages":T33, "PDP"=w218:T34, "Channel Content"=→"What's connected?":string)  [unwired: 8 in, 1 out]
        n99 = Bundle("Numeric"=w182, "Numeric"=w181) -> (→"Chart 2":cluster{"Numeric":dbl, "Numeric":dbl})  [unwired: 1 in]
        n100 = call "pneumatics.vi"("Enable Compressor"="Enable Compressor") -> ()  [unwired: 3 in]
        n101 = call "leds.vi"("LED Robot Mode"="LED Robot Mode", "Opening Ceremonies Mode"="Opening Ceremonies Mode", "Override?"="Override LED Mode", "LEDs Off?"="LEDs OFF") -> ()
        n102 = Unbundle(w218) -> ("all currents (A)"=→"All Currents (A)":dbl[], "PDP Energy"=→"PDP Energy":cluster{"Energy (J)":dbl, "Power (W)":dbl}, "voltage (V)"=→"Voltage":dbl, "temperature (F)"=→"Temperature":dbl, "current (A)"=→"Current":dbl)
        n103 = call "settings.vi"("refresh"="refresh", "Update"="update", "New Values"="Values") -> ("Values"=w194:string[], "Keys"=→"Keys":string[], "Refresh?"=w195:bool)  [unwired: 6 in]
        n104 = case shown="True" w195 {
          tunnel: w194 -> [_ w222]
          frame False {
          }
          frame True {
            n105 = local write "Values"(w222) -> ()
          }
        }
      }
    }
    "Robot Connection" <- w168
    n106 = local read "Code?"() -> (w166:enum16{"unknown", "noCode", "code"})
    n107 = Equal?(x=enum16{"unknown", "noCode", "code"}."code", y=w166) -> (x = y?=w164:bool)
    n108 = And(x=w163, y=w164) -> (x .and. y?=→"Dashboard Connection":bool)
    n109 = Wait (ms)(milliseconds to wait=u32 100) -> ()  [unwired: 1 out]
    "Dashboard Revision" <- w161
  }
  n110 = while {
    stop <- FALSE stop-if-true
    w232 = T35 {"Safety Data Prev Iteration"=[], "Item Names"=[]} ("Safety Data and Log")
    # "Safeties"
    # "fast loop"
    # "Clock"
    n111 = local read "Reset Error Log"() -> (w229:bool)
    n112 = feedback #1(w232) -> (w230:T35)
    n113 = Select(t=w232, s=w229, f=w230) -> (s? t:f=w231:T35)
    n114 = call "safeties.vi"("Prev Iteration Data"=w231) -> ("Safety Data and Log"=w228:T35, "Shooter"=→"Shooter":T10, "Ramp Belts"=→"Ramp Belts":T9, "Arm Actuator"=→"Arm Actuator":T8, "Drive Train"=→"Drive Train":T7)  [unwired: 6 in]
    n115 = feedback-in #1(w228) -> ()
    n116 = Unbundle(w228) -> ("Item Names"=w227:string[][])  [unwired: 1 out]
    n117 = Get Date/Time String(date format (0)=enum16{"short", "long", "abbreviated"}."short", want seconds? (F)=FALSE) -> (date string=w237:string, time string=w238:string)  [unwired: 1 in]
    n118 = property on="Error Log" class="MCListbox (strict)"("ItemNames"=w227) -> ()  [unwired: 2 in, 2 out]
    n119 = Concatenate Strings(w237, "                  ", w238) -> (→"Time":string)
    n120 = disable-structure shown="Enabled" {
      frame Disabled {
        # "auto info"
        n121 = local read item#-1() -> ()  [unwired: 1 out]
        n122 = call "auto info.vi"() -> ("About Selected Auto Mode"=→"About Selected Auto Mode":string)  [unwired: 1 in]
      }
      frame Enabled {
      }
    }
    n123 = case shown="True" "Reset Error Log" {
      frame False {
      }
      frame True {
        n124 = property on="Error Log" class="MCListbox (strict)"("ItemNames"=string[][] [] ("Item Names")) -> ()  [unwired: 2 in, 2 out]
      }
    }
    n125 = Wait (ms)(milliseconds to wait=u32 20) -> ()  [unwired: 1 out]
  }
  n126 = call "IMAQ Create"("Image Name"="Dashboard Image", "Image Type"=w7) -> ("New Image"=w5:T6, "error out"=w6:errorcluster)  [unwired: 2 in, 1 out]
  n127 = property on="Camera Settings" class="Clust (strict)"("Visible"=w1) -> ()  [unwired: 2 in, 2 out]
  n128 = local write "DB Camera Config"(w1) -> ()
  n129 = while {
    tunnel: w5 -> [w258]
    tunnel: w6 -> [_]
    tunnel: [w259] -> _
    i -> [w259]
    stop <- FALSE stop-if-true
    w244 = u16 2 items=["Camera Off", "USB Camera SW", "USB Camera HW", "IP Camera"] ("Camera Mode")
    w245 = u16 3 items=["Camera Off", "USB Camera SW", "USB Camera HW", "IP Camera"] ("Camera Mode")
    # "hidden/disabled"
    # "Optionally read the DB image,\nlog, or retrieve images from a\nlogged match"
    n130 = call-poly <vilib>:"NT Read Value.vi"("Name"="camera_override") -> ("Boolean"=w249:bool)  [unwired: 9 in, 1 out]
    "Camera In Targeting Mode" <- w249
    n131 = Select(t=w249, s=w249, f="Camera Selector") -> (s? t:f=w247:bool)
    "Shooter Camera Active" <- w247
    n132 = Not(x=w247) -> (.not. x?=→"Intake Camera Active":bool)
    n133 = Select(t=w245, s=w247, f=w244) -> (s? t:f=w246:u16)
    n134 = local read "Rec Mode"() -> (w253:enum32{"Stop", "Record", "Playback"})
    n135 = local read "Camera IP"() -> (w261:string)
    n136 = call <vilib>:"WPI_CameraRead MJPG for Dashboard.vi"("Camera Settings"="Camera Settings", "Rec Mode"=w253, "Camera IP"=w261, "Camera Mode"=w246, "Refnum in"=w258) -> ("Active"=w256:bool, "Refnum out"=w257:T6, "FPS"=w255:dbl, "Bandwidth (Mbps)"=w254:dbl)  [unwired: 3 in]
    n137 = case shown="True" w256 {
      tunnel: w257 -> [_ w292]
      tunnel: w254 -> [_ w291]
      tunnel: w255 -> [_ w290]
      frame False {
        # "Sleep for 500ms"
        n138 = Wait Until Next ms Multiple(millisecond multiple=u32 500) -> ()  [unwired: 1 out]
      }
      frame True {
        w281 = u16 1 items=["RGB", "HSL", "HSV", "HSI"] ("Color Mode")
        w285 = T22 4 items=["Grayscale (U8)", "Grayscale (I16)", "Grayscale (SGL)", "Complex (CSG)", "RGB (U32)", "HSL (U32)", "RGB (U64)", "Grayscale (U16)"] ("Image Type")
        # "Update Mbps LED"
        n139 = call "IMAQ Clear Overlay"("Image"=w292) -> ("error out"=w295:errorcluster, "Image Out"=w283:T6)  [unwired: 2 in, 7 out]
        "Camera Image" <- w283
        "Image" <- w283
        n140 = To Long Integer(number=w291) -> (32bit integer=w288:i32)
        "Mbps" <- w288
        n141 = Unbundle By Name(w295) -> ("status"=w296:bool)
        n142 = case shown="Default" w288 {
          tunnel: [u32 6618880 ("Color Box") u32 16776722 ("Color Box") u32 16716800 ("Color Box")] -> w293
          frame Default {
          }
          frame 4, 5 {
          }
          frame 6.. {
          }
        }
        n143 = property on="Image Message" class="Str"("Visible"=w296) -> ()  [unwired: 2 in, 2 out]
        n144 = Bundle("Color Box"=w293, "Color Box"=w293) -> (w294:cluster{"Color Box":u32, "Color Box":u32})  [unwired: 1 out]
        n145 = Build Array(w294) -> (w289:cluster{"Color Box":u32, "Color Box":u32}[])
        n146 = property on="Mbps 2" class="Bool (strict)"("Colors [4]"=w289) -> ()  [unwired: 2 in, 2 out]
        n147 = call "IMAQ Create"("Image Name"="processed", "Image Type"=w285) -> ("New Image"=w286:T6, "error out"=w282:errorcluster)  [unwired: 3 in]
        n148 = call "IMAQ Copy"("error in (no error)"=w282, "Image Dst"=w286, "Image Src"=w283) -> ("error out"=w264:errorcluster, "Image Dst Out"=w277:T6)  [unwired: 3 in]
        n149 = call "IMAQ ColorThreshold"("Blue or Luma or Val or Inten Range"="Luma Range", "Replace Value"=1, "Green or Sat Range"="Sat Range", "Color Mode"=w281, "error in (no error)"=w264, "Red or Hue Range"="Hue Range", "Image Src"=w277) -> ("error out"=w265:errorcluster, "Image Dst Out"=w278:T6)  [unwired: 3 in]
        n150 = call "IMAQ FillHole"("error in (no error)"=w265, "Image Src"=w278) -> ("error out"=w266:errorcluster, "Image Dst Out"=w275:T6)  [unwired: 4 in]
        n151 = call "IMAQ RemoveParticle"("Connectivity 4/8 (8)"=TRUE, "Low Pass/High Pass (Low)"=FALSE, "Square/Hexa (Square)"=FALSE, "error in (no error)"=w266, "Number of Erosion"=1, "Image Src"=w275) -> ("error out"=w267:errorcluster, "Image Dst Out"=w270:T6)  [unwired: 1 in, 3 out]
        n152 = call "IMAQ Convex Hull"("error in (no error)"=w267, "Image Src"=w270) -> ("error out"=w268:errorcluster, "Image Dst Out"=w269:T6)  [unwired: 8 in]
        n153 = call "vision process goal.vi"(8:w268, "Processed Image"=w269) -> ("Annotated Image Out"=→"Targets":T6)  [unwired: 8 in, 1 out]
        "fps" <- w290
      }
    }
  }
  n154 = property on="hover hint" class="Str"("Visible"=TRUE) -> ()  [unwired: 2 in, 2 out]
  n155 = disable-structure shown="Disabled" {
    frame Disabled {
      (unwired) 0.0 ("temperature")
      w304 = enum32{"Stop", "Record", "Playback"}."Stop" ("Rec Mode")
      w300 = FALSE ("Visible")
      # "Basic debug and auto controls: Their data names are fixed, but\nthe displayed name, called a caption, can be changed directly or in\nrobot code such as shown in Begin."
      # "Additional UI Initialization"
      # "Controls for Test Mode, Camera Settings, etc."
      # "Loop 6. Animation for background of window during playback and record"
      # "Loop 4. Process UI events related to test mode, checklist, and camera settings"
      n156 = property class="VI" props=["Front Panel.Closeable"]() -> (reference out=w303:refnum<vi>)  [unwired: 2 in, 2 out]
      n157 = property class="VI"() -> ("Panel"=w306:refnum<vi>)  [unwired: 2 in, 2 out]
      n158 = control-ref of="CheckList"() -> (w302:refnum<vi>)
      n159 = register-events(refnum<vi> refnum) -> (reference out=w312:refnum<event-registration>, error out=w313:errorcluster)  [unwired: 2 in]
      n160 = property class="Pnl"(reference=w306) -> ("Panes[]"=w305:refnum<vi>[])  [unwired: 1 in, 2 out]
      n161 = vi-ref "Playback Controls.vi"() -> (w311:refnum<vi>)
      n162 = call "Initialize Camera and CheckList.vi"("ListBox in"=w302) -> ("Cluster"=w301:cluster{"value":i32, "value":i32, "index":i32}, "Array"=w308:cluster{string[]}[], "File Refnum"=w309:T40)  [unwired: 8 in]
      n163 = Index Array(array=w305) -> (element=w307:refnum<vi>)  [unwired: 1 in]
      n164 = while {
        tunnel: w307 -> [w316]
        i -> [w319]
        stop <- FALSE stop-if-true
        n165 = Wait (ms)(milliseconds to wait=u32 100) -> ()  [unwired: 1 out]
        n166 = case shown="\"Stop\", Default" "Rec Mode" {
          tunnel: w319 -> [_ _ w334]
          tunnel: [u32 2829099 ("Base Color") u32 11141120 ("Target Color") w323] -> w315
          frame "Stop", Default {
            # "Reset the color, extra updates don't cost much"
          }
          frame "Record" {
          }
          frame "Playback" {
            # "Playback"
            n167 = Quotient & Remainder(x=w334, y=u32 50 ("milliseconds to wait")) -> (x-y*floor(x/y)=w330:u32)  [unwired: 1 out]
            n168 = Divide(x=w330, y=u32 50 ("milliseconds to wait")) -> (x/y=w327:dbl)
            n169 = Multiply(x=6.283185307179586, y=w327) -> (x*y=w332:dbl)
            n170 = Sine(x=w332) -> (sin(x)=w331:dbl)
            n171 = Absolute Value(x=w331) -> (abs(x)=w324:dbl)
            n172 = call "Interpolate RGB Color.vi"("Proportion"=w324, "Target Color"=u32 30976, "Base Color"=u32 2829099) -> ("Result Color"=w323:u32)  [unwired: 8 in]
          }
        }
        n173 = property class="Pane"(reference=w316, "PaneColor"=w315) -> ()  [unwired: 1 in, 2 out]
      }
      n174 = control-ref of="Test Tree"() -> (w310:refnum<vi>)
      n175 = while {
        tunnel: w308 -> [w342]
        shift-right: [w341] -> _
        shift-left: w309 -> [w340]
        tunnel: [w339] -> _
        tunnel: w310 -> [w338]
        tunnel: w311 -> [w337]
        tunnel: w312 -> [w336]
        tunnel: w313 -> [_]
        tunnel: w303 -> [w335]
        i -> [w339]
        stop <- FALSE stop-if-true
        n176 = event shown="[0] Timeout" {
          selector: w336 -> [_ _ _ _ _ _ _ _ _ _ _ _ _ _ _ _ _]
          dyn-events: [_ _ _ _ _ _ _ _ _ _ _ _ _ w578 _ _ _] -> _
          timeout: u32 60 ("milliseconds to wait") -> [_ _ _ _ _ _ _ _ _ _ _ _ _ _ _ _ _]
          tunnel: w338 -> [w354 _ _ _ _ _ _ _ _ _ _ _ _ _ _ _ _]
          tunnel: "Test Tree" -> [_ _ _ _ _ _ _ _ w547 w555 w557 w561 w569 _ _ _ _]
          tunnel: w342 -> [_ w374 _ _ _ _ w511 w542 _ _ _ _ _ _ _ _ _]
          tunnel: [w350 w373 w472 w477 w485 w497 w510 w535 w546 w553 w556 w560 w568 w580 w594 w595 w605] -> w341
          tunnel: w340 -> [w350 w373 w472 w477 w485 w497 w509 w535 w546 w553 w556 w560 w568 w580 w594 w595 w605]
          tunnel: w337 -> [_ _ _ _ _ _ _ _ _ _ _ _ _ w581 _ w598 _]
          tunnel: w335 -> [_ _ _ _ _ _ _ _ _ _ _ _ _ w576 _ _ _]
          event Timeout {
            n177 = event-data() -> ()  [unwired: 1 in, 1 out]
            n178 = local read "Robot Mode"() -> (w353:T2)
            n179 = Index Array(array=T36 [{"Operation"=enum."Clear", "Color Box"=14013909}, {"Operation"=enum."Clear", "Color Box"=14013909}, {"Operation"=enum."Clear", "Color Box"=14013909}, {"Operation"=enum."Clear", "Color Box"=14013909}, {"Operation"=enum."Update", "Color Box"=14013909}, {"Operation"=enum."Update", "Color Box"=16777215}, {"Operation"=enum."Clear", "Color Box"=14013909}, {"Operation"=enum."Clear", "Color Box"=14013909}, {"Operation"=enum."Clear", "Color Box"=14013909}], index=w353) -> (element=w348:T41)
            n180 = Unbundle(w348) -> ("Operation"=w347:enum16{"Update", "Clear"}, "Color Box"=w346:u32)
            n181 = call <vilib>:"NT Read String.vi"("Name"="TestMode/TestName") -> ("String"=w357:string)  [unwired: 9 in, 1 out]
            n182 = case shown="\"Data\"" "Dashboard Tab" {
              tunnel: w354 -> [_ w365 _]
              tunnel: "/TestMode/Automatic/" ("Name Pattern") -> [_ w364 _]
              tunnel: w347 -> [_ w363 _]
              tunnel: w346 -> [_ w359 _]
              frame "Data", Default {
              }
              frame "Data" {
                w362 = -2 ("Active Item:Row Number")
                n183 = call <vilib>:"NT Read and Format Entries as Tree.vi"("Operation"=w363, "Name Pattern"=w364, "Tree Refnum"=w365) -> ()  [unwired: 7 in, 2 out]
                n184 = property on="Test Tree" class="Tree (strict)"("Active Item Row Number"=w362, "ActiveColNum"=w362, "CellBG"=w359, "Active Item Row Number"=-1 ("Active Item:Row Number"), "CellBG"=u32 5789784 ("Color Box")) -> ()  [unwired: 2 in, 2 out]
              }
              frame "Network Variables" {
              }
            }
            n185 = case shown="\"\"" w357 {
              tunnel: "TestMode/TestProgress" ("Name") -> [w367 _]
              tunnel: "TestMode/TestProgressText" ("Name") -> [w366 _]
              frame Default {
                n186 = call <vilib>:"NT Read Number.vi"("Name"=w367) -> ("Numeric"=w368:dbl)  [unwired: 9 in, 1 out]
                n187 = call <vilib>:"NT Read String.vi"("Name"=w366) -> ("String"=w369:string)  [unwired: 9 in, 1 out]
                n188 = Bundle("Numeric"=w368, "String"=w369) -> (→"Progress":cluster{"Numeric":dbl, "String":string})  [unwired: 1 in]
              }
              frame "" {
                n189 = property on="Progress" class="Clust (strict)"("Visible"=FALSE) -> ()  [unwired: 2 in, 2 out]
                n190 = local write "Test Name"(u16 0) -> ()
              }
            }
          }
          event "Test Tree": Value Change {
            # "Show appropriate\ncontrols"
            n191 = event-data() -> ("CtlRef"=w377:refnum<vi>, "NewVal"=w375:string)  [unwired: 1 in]
            n192 = call <vilib>:"WPI_UtilitiesGetTreeIOName.vi"("NewVal"=w375, "TreeControl in"=w377) -> ("I/O Name"=w378:string)  [unwired: 9 in]
            n193 = case shown="\"Motor\", \"PWM\"" w378 {
              selector: w378 -> [_ w385 _ w403 w412 _]
              tunnel: w375 -> [_ _ w400 w402 _ w419]
              tunnel: w374 -> [_ _ _ _ _ w418]
              frame Default {
                w380 = FALSE ("Visible")
                w379 = FALSE ("Visible")
                n194 = property on="Motor" class="Clust (strict)"("Visible"=w379) -> ()  [unwired: 2 in, 2 out]
                n195 = property on="Test Ring" class="Ring (strict)"("Visible"=w379) -> ()  [unwired: 2 in, 2 out]
                n196 = property on="Rev/Fwd" class="Clust (strict)"("Visible"=w380) -> ()  [unwired: 2 in, 2 out]
                n197 = property on="On/Off" class="Bool (strict)"("Visible"=w380) -> ()  [unwired: 2 in, 2 out]
                n198 = property on="Test Slider" class="Slide (strict)"("Visible"=w380) -> ()  [unwired: 2 in, 2 out]
              }
              frame "Motor", "PWM" {
                w386 = FALSE ("Visible")
                n199 = case shown="\"Motor\", Default" w385 {
                  tunnel: [1.0 ("Value") -1.0 ("Value")] -> w384
                  tunnel: [255.0 ("Value") 1.0 ("Value")] -> w383
                  tunnel: [128.0 ("Value") 0.0 ("Value")] -> w382
                  tunnel: [64.0 ("Value") 0.5 ("Value")] -> w381
                  frame "PWM" {
                  }
                  frame "Motor", Default {
                  }
                }
                n200 = property on="Motor" class="Clust (strict)"("Visible"=TRUE) -> ()  [unwired: 2 in, 2 out]
                n201 = property on="Value" class="Slide (strict)"("Value"=w382, "Scale.Minimum"=w384, "Scale.Maximum"=w383, "Scale.Increment"=w381) -> ()  [unwired: 2 in, 2 out]
                n202 = property on="On/Off" class="Bool (strict)"("Visible"=w386) -> ()  [unwired: 2 in, 2 out]
                n203 = property on="Test Slider" class="Slide (strict)"("Visible"=w386) -> ()  [unwired: 2 in, 2 out]
                n204 = property on="Test Ring" class="Ring (strict)"("Visible"=w386) -> ()  [unwired: 2 in, 2 out]
                n205 = property on="Rev/Fwd" class="Clust (strict)"("Visible"=w386) -> ()  [unwired: 2 in, 2 out]
              }
              frame "Servo" {
                w398 = FALSE ("Visible")
                n206 = call <vilib>:"NT Read Number.vi"("Name"=w400) -> ("Numeric"=w399:dbl)  [unwired: 9 in, 1 out]
                n207 = property on="Test Slider" class="Slide (strict)"("Visible"=TRUE, "Scale.Maximum"=170.0 ("Scale.Range:Maximum")) -> ()  [unwired: 2 in, 2 out]
                n208 = local write "Test Slider"(w399) -> ()
                n209 = property on="Motor" class="Clust (strict)"("Visible"=w398) -> ()  [unwired: 2 in, 2 out]
                n210 = property on="Rev/Fwd" class="Clust (strict)"("Visible"=w398) -> ()  [unwired: 2 in, 2 out]
                n211 = property on="On/Off" class="Bool (strict)"("Visible"=w398) -> ()  [unwired: 2 in, 2 out]
                n212 = property on="Test Ring" class="Ring (strict)"("Visible"=w398) -> ()  [unwired: 2 in, 2 out]
              }
              frame "Relay", "Solenoid" {
                w401 = FALSE ("Visible")
                n213 = property on="Motor" class="Clust (strict)"("Visible"=w401) -> ()  [unwired: 2 in, 2 out]
                n214 = property on="Test Slider" class="Slide (strict)"("Visible"=w401) -> ()  [unwired: 2 in, 2 out]
                n215 = Search and Replace String(input string=w402, search string="/Value  **", replace string="/Direction") -> (result string=w408:string)  [unwired: 5 in, 3 out]
                n216 = property on="Test Ring" class="Ring (strict)"("Visible"=w401) -> ()  [unwired: 2 in, 2 out]
                n217 = call <vilib>:"NT Read String.vi"("Name"=w408) -> ("String"=w406:string)  [unwired: 9 in, 1 out]
                n218 = Equal?(x="Both directions", y=w406) -> (x = y?=w404:bool)
                n219 = Not(x=w404) -> (.not. x?=w405:bool)
                n220 = property on="Rev/Fwd" class="Clust (strict)"("Visible"=w404) -> ()  [unwired: 2 in, 2 out]
                n221 = property on="On/Off" class="Bool (strict)"("Visible"=w405, "Caption.Text"=w403) -> ()  [unwired: 2 in, 2 out]
              }
              frame "Compressor", "Digital Out" {
                w411 = FALSE ("Visible")
                # "Get direction and finish"
                n222 = property on="Motor" class="Clust (strict)"("Visible"=w411) -> ()  [unwired: 2 in, 2 out]
                n223 = property on="Test Slider" class="Slide (strict)"("Visible"=w411) -> ()  [unwired: 2 in, 2 out]
                n224 = property on="Test Ring" class="Ring (strict)"("Visible"=w411) -> ()  [unwired: 2 in, 2 out]
                n225 = property on="On/Off" class="Bool (strict)"("Visible"=TRUE, "Caption.Text"=w412) -> ()  [unwired: 2 in, 2 out]
                n226 = property on="Rev/Fwd" class="Clust (strict)"("Visible"=FALSE) -> ()  [unwired: 2 in, 2 out]
              }
              frame "Camera" {
                n227 = call <vilib>:"Get Last Path Segment.vi"("String in"=w419) -> ("String out"=w420:string)  [unwired: 10 in]
                n228 = property on="On/Off" class="Bool (strict)"("Visible"=FALSE) -> ()  [unwired: 2 in, 2 out]
                n229 = property on="Motor" class="Clust (strict)"("Visible"=FALSE) -> ()  [unwired: 2 in, 2 out]
                n230 = property on="Rev/Fwd" class="Clust (strict)"("Visible"=FALSE) -> ()  [unwired: 2 in, 2 out]
                n231 = case shown="\"Exposure Priority  **\"" w420 {
                  tunnel: w419 -> [w426 w435 w444 w453 w462 _ w468]
                  tunnel: w418 -> [w424 w432 w441 w450 w459 _ _]
                  frame "Size  **" {
                    n232 = Index Array(array=w424) -> (element=w423:cluster{string[]})  [unwired: 1 in]
                    n233 = call <vilib>:"NT Read String.vi"("Name"=w426) -> ("String"=w425:string)  [unwired: 9 in, 1 out]
                    n234 = Unbundle(w423) -> (w421:string[])
                    n235 = Match First String(2:w421, 3:w425) -> (0:w422:i32)  [unwired: 1 out]
                    n236 = property on="Test Ring" class="Ring (strict)"("Value"=w422, "Strings []"=w421) -> ()  [unwired: 2 in, 2 out]
                    n237 = property on="Test Ring" class="Ring (strict)"("Visible"=TRUE) -> ()  [unwired: 2 in, 2 out]
                    n238 = property on="Test Slider" class="Slide (strict)"("Visible"=FALSE) -> ()  [unwired: 2 in, 2 out]
                  }
                  frame "White Balance  **" {
                    n239 = Index Array(array=w432, index=1) -> (element=w433:cluster{string[]})
                    n240 = call <vilib>:"NT Read String.vi"("Name"=w435) -> ("String"=w434:string)  [unwired: 9 in, 1 out]
                    n241 = Unbundle(w433) -> (w430:string[])
                    n242 = Match First String(2:w430, 3:w434) -> (0:w429:i32)  [unwired: 1 out]
                    n243 = property on="Test Ring" class="Ring (strict)"("Value"=w429, "Strings []"=w430) -> ()  [unwired: 2 in, 2 out]
                    n244 = property on="Test Ring" class="Ring (strict)"("Visible"=TRUE) -> ()  [unwired: 2 in, 2 out]
                    n245 = property on="Test Slider" class="Slide (strict)"("Visible"=FALSE) -> ()  [unwired: 2 in, 2 out]
                  }
                  frame "Exposure  **" {
                    n246 = Index Array(array=w441, index=2) -> (element=w442:cluster{string[]})
                    n247 = call <vilib>:"NT Read String.vi"("Name"=w444) -> ("String"=w443:string)  [unwired: 9 in, 1 out]
                    n248 = Unbundle(w442) -> (w438:string[])
                    n249 = Match First String(2:w438, 3:w443) -> (0:w439:i32)  [unwired: 1 out]
                    n250 = property on="Test Ring" class="Ring (strict)"("Value"=w439, "Strings []"=w438) -> ()  [unwired: 2 in, 2 out]
                    n251 = property on="Test Ring" class="Ring (strict)"("Visible"=TRUE) -> ()  [unwired: 2 in, 2 out]
                    n252 = property on="Test Slider" class="Slide (strict)"("Visible"=FALSE) -> ()  [unwired: 2 in, 2 out]
                  }
                  frame "Exposure Priority  **" {
                    n253 = Index Array(array=w450, index=3) -> (element=w451:cluster{string[]})
                    n254 = call <vilib>:"NT Read String.vi"("Name"=w453) -> ("String"=w452:string)  [unwired: 9 in, 1 out]
                    n255 = Unbundle(w451) -> (w447:string[])
                    n256 = Match First String(2:w447, 3:w452) -> (0:w448:i32)  [unwired: 1 out]
                    n257 = property on="Test Ring" class="Ring (strict)"("Value"=w448, "Strings []"=w447) -> ()  [unwired: 2 in, 2 out]
                    n258 = property on="Test Ring" class="Ring (strict)"("Visible"=TRUE) -> ()  [unwired: 2 in, 2 out]
                    n259 = property on="Test Slider" class="Slide (strict)"("Visible"=FALSE) -> ()  [unwired: 2 in, 2 out]
                  }
                  frame "Color Enable  **" {
                    n260 = Index Array(array=w459, index=4) -> (element=w460:cluster{string[]})
                    n261 = call <vilib>:"NT Read String.vi"("Name"=w462) -> ("String"=w461:string)  [unwired: 9 in, 1 out]
                    n262 = Unbundle(w460) -> (w456:string[])
                    n263 = Match First String(2:w456, 3:w461) -> (0:w457:i32)  [unwired: 1 out]
                    n264 = property on="Test Ring" class="Ring (strict)"("Value"=w457, "Strings []"=w456) -> ()  [unwired: 2 in, 2 out]
                    n265 = property on="Test Ring" class="Ring (strict)"("Visible"=TRUE) -> ()  [unwired: 2 in, 2 out]
                    n266 = property on="Test Slider" class="Slide (strict)"("Visible"=FALSE) -> ()  [unwired: 2 in, 2 out]
                  }
                  frame Default {
                    n267 = property on="Test Ring" class="Ring (strict)"("Visible"=FALSE) -> ()  [unwired: 2 in, 2 out]
                    n268 = property on="Test Slider" class="Slide (strict)"("Visible"=FALSE) -> ()  [unwired: 2 in, 2 out]
                  }
                  frame "Brightness  **", "Color Level  **", "Compression  **", "FPS  **", "Sharpness  **" {
                    n269 = call <vilib>:"NT Read Number.vi"("Name"=w468) -> ("Numeric"=w467:dbl)  [unwired: 9 in, 1 out]
                    n270 = local write "Test Slider"(w467) -> ()
                    n271 = property on="Test Slider" class="Slide (strict)"("Visible"=TRUE, "Scale.Maximum"=100.0 ("Scale.Range:Maximum")) -> ()  [unwired: 2 in, 2 out]
                    n272 = property on="Test Ring" class="Ring (strict)"("Visible"=FALSE) -> ()  [unwired: 2 in, 2 out]
                  }
                }
              }
            }
            n273 = property on="Progress" class="Clust (strict)"("Visible"=FALSE) -> ()  [unwired: 2 in, 2 out]
          }
          event "Test Name": Mouse Enter {
            # "Populate the ring with the list of tests"
            n274 = event-data() -> ()  [unwired: 1 in, 1 out]
            n275 = call <vilib>:"NT Read String Array.vi"("Name"="TestMode/TestList") -> ("String Array"=w476:string[])  [unwired: 9 in, 1 out]
            n276 = Build Array (concatenate)("Select the test to run...", w476) -> (w475:string[])
            n277 = property on="Test Name" class="Ring (strict)"("Strings []"=w475) -> ()  [unwired: 2 in, 2 out]
          }
          event "Test Name": Value Change {
            w478 = FALSE ("Visible")
            # "Tell the robot the test name to run"
            n278 = event-data() -> ("NewVal"=w482:u16)  [unwired: 1 in]
            n279 = property on="Test Name" class="Ring (strict)"() -> ("Strings []"=w483:string[])  [unwired: 2 in, 2 out]
            n280 = local write "Progress"(T3 {"Test Progress"=0, "Test Progress Text"=""} ("Progress")) -> ()
            n281 = Index Array(array=w483, index=w482) -> (element=w481:string)
            n282 = call <vilib>:"NT Write String.vi"("String"=w481, "Name"="TestMode/TestName") -> ()  [unwired: 9 in, 1 out]
            n283 = property on="Progress" class="Clust (strict)"("Visible"=TRUE) -> ()  [unwired: 2 in, 2 out]
            n284 = property on="Motor" class="Clust (strict)"("Visible"=w478) -> ()  [unwired: 2 in, 2 out]
            n285 = property on="Test Slider" class="Slide (strict)"("Visible"=w478) -> ()  [unwired: 2 in, 2 out]
            n286 = property on="On/Off" class="Bool (strict)"("Visible"=w478) -> ()  [unwired: 2 in, 2 out]
            n287 = property on="Rev/Fwd" class="Clust (strict)"("Visible"=w478) -> ()  [unwired: 2 in, 2 out]
            n288 = property on="Test Ring" class="Ring (strict)"("Visible"=w478) -> ()  [unwired: 2 in, 2 out]
          }
          event "Listbox": Double Click {
            # "Shift clears all"
            # "Update symbols on the listbox"
            n289 = event-data() -> ("PlatMods.Shift"=w486:bool, "Row"=w488:i32)  [unwired: 1 in]
            n290 = case shown="True" w486 {
              tunnel: w488 -> [w492 _]
              tunnel: 1 -> [w491 _]
              frame False {
                n291 = property on="Listbox" class="LstBox (strict)"() -> ("Item Symbols"=w490:i32[])  [unwired: 2 in, 2 out]
                n292 = Replace Array Subset(array=w490, new element=w491, index=w492) -> (w489:i32[])
                n293 = property on="Listbox" class="LstBox (strict)"("Item Symbols"=w489) -> ()  [unwired: 2 in, 2 out]
              }
              frame True {
                w493 = 0 ("Top Row")
                n294 = property on="Listbox" class="LstBox (strict)"() -> ("Number of Rows"=w495:u32)  [unwired: 2 in, 2 out]
                n295 = Initialize Array(0, w495) -> (w494:i32[])
                n296 = property on="Listbox" class="LstBox (strict)"("Top Row"=w493, "Value"=w493, "Item Symbols"=w494) -> ()  [unwired: 2 in, 2 out]
              }
            }
          }
          event "Listbox": Key Down {
            # "Update symbols on the listbox\nLeft and right keys check and uncheck"
            n297 = event-data() -> ("VKey"=w499:T37)  [unwired: 1 in]
            n298 = case shown="\"Left\", \"Right\"" w499 {
              selector: w499 -> [w504 _]
              tunnel: eventvkey."Left" ("VKey") -> [w502 _]
              frame "Left", "Right" {
                n299 = Equal?(x=w502, y=w504) -> (x = y?=w503:bool)
                n300 = Select(t=0, s=w503, f=1) -> (s? t:f=w505:i32)
                n301 = property on="Listbox" class="LstBox (strict)"() -> ("Item Symbols"=w508:i32[])  [unwired: 2 in, 2 out]
                n302 = Replace Array Subset(array=w508, new element=w505, index="Listbox") -> (w507:i32[])
                n303 = property on="Listbox" class="LstBox (strict)"("Item Symbols"=w507) -> ()  [unwired: 2 in, 2 out]
              }
              frame Default {
              }
            }
          }
          event "DB Camera Config": Value Change {
            # "Show or hide the cluster of controls, store in ini file"
            n304 = event-data() -> ("NewVal"=w512:bool)  [unwired: 1 in]
            n305 = case shown="False" w512 {
              tunnel: w511 -> [w522 _]
              tunnel: [w515 w533] -> w510
              tunnel: w509 -> [w514 w533]
              frame False {
                w529 = "Camera"
                w513 = FALSE ("Visible")
                n306 = local read "Camera Settings"() -> (w521:T5)
                n307 = Index Array(array=w522) -> (element=w525:cluster{string[]})  [unwired: 1 in]
                n308 = Unbundle(w521) -> ("Frame Rate"=w520:i32, "Compression"=w519:i32, "Size"=w523:u16)
                n309 = Unbundle(w525) -> (w524:string[])
                n310 = Index Array(array=w524, index=w523) -> (element=w518:string)
                n311 = call-poly <vilib>:"Write Key.vi"("section"=w529, "value"=w518, "key"="Size", "refnum"=w514) -> ("refnum out"=w531:T40)  [unwired: 2 in, 5 out]
                n312 = call-poly <vilib>:"Write Key.vi"("section"=w529, "value"=w520, "key"="FrameRate", "refnum"=w531) -> ("refnum out"=w530:T40)  [unwired: 1 in, 6 out]
                n313 = local write "DB Camera Config"(w513) -> ()
                n314 = call-poly <vilib>:"Write Key.vi"("section"=w529, "value"=w519, "key"="Compression", "refnum"=w530) -> ("refnum out"=w516:T40)  [unwired: 1 in, 6 out]
                n315 = property on="Camera Settings" class="Clust (strict)"("Visible"=w513) -> ()  [unwired: 2 in, 2 out]
                n316 = call <vilib>:"Close Config Data.vi"("refnum"=w516) -> ("file path"=w517:path)  [unwired: 2 in, 8 out]
                n317 = call <vilib>:"Open Config Data.vi"("configuration file path"=w517) -> ("refnum"=w515:T40)  [unwired: 8 in, 2 out]
              }
              frame True {
                n318 = property on="Camera Settings" class="Clust (strict)"("Visible"=TRUE) -> ()  [unwired: 2 in, 2 out]
              }
            }
          }
          event "Camera Settings": Value Change {
            # "Update summary string when any elements of DB camera change"
            n319 = event-data() -> ("NewVal"=w545:T5)  [unwired: 1 in]
            n320 = Index Array(array=w542) -> (element=w541:cluster{string[]})  [unwired: 1 in]
            n321 = Unbundle(w545) -> ("Frame Rate"=w537:i32, "Compression"=w536:i32, "Size"=w539:u16)
            n322 = Unbundle(w541) -> (w540:string[])
            n323 = Index Array(array=w540, index=w539) -> (element=w538:string)
            n324 = Format Into String(format string="%s   %dfps   %d%%", w538, w537, w536) -> (resulting string=w543:string)  [unwired: 2 in, 1 out]
            n325 = Build Array(w543) -> (w534:string[])
            n326 = property on="DB Camera Config" class="Bool (strict)"("Strings [4]"=w534) -> ()  [unwired: 2 in, 2 out]
          }
          event "Motor.Enable": Value Change {
            # "When the test mode otor enable helper is set, update that\ntree row item's value"
            n327 = event-data() -> ("NewVal"=w551:bool)  [unwired: 1 in]
            n328 = Unbundle("Motor") -> ("Value"=w550:dbl)  [unwired: 1 out]
            n329 = Select(t=w550, s=w551, f=0.0) -> (s? t:f=w548:dbl)
            n330 = call <vilib>:"NT Write Number.vi"("Numeric"=w548, "Name"=w547) -> ()  [unwired: 9 in, 1 out]
          }
          event "Test Slider": Value Change {
            # "When the test mode slider helper is set, update that\ntree row item's value"
            n331 = event-data() -> ("NewVal"=w554:dbl)  [unwired: 1 in]
            n332 = call <vilib>:"NT Write Number.vi"("Numeric"=w554, "Name"=w555) -> ()  [unwired: 9 in, 1 out]
          }
          event "On/Off": Value Change {
            # "When the test mode on/off helper value is set, update that\ntree row item's value"
            n333 = event-data() -> ("NewVal"=w559:bool)  [unwired: 1 in]
            n334 = Boolean To (0,1)(Boolean=w559) -> (0, 1=w558:i16)
            n335 = call <vilib>:"NT Write Number.vi"("Numeric"=w558, "Name"=w557) -> ()  [unwired: 9 in, 1 out]
          }
          event "Rev/Fwd": Value Change {
            # "When the test mode helper value for relays is set, update that\ntree row item's value"
            n336 = event-data() -> ("NewVal.Forward"=w567:bool, "NewVal.Reverse"=w566:bool)  [unwired: 1 in]
            n337 = Boolean To (0,1)(Boolean=w567) -> (0, 1=w563:i16)
            n338 = Boolean To (0,1)(Boolean=w566) -> (0, 1=w565:i16)
            n339 = Negate(x=w565) -> (-x=w564:i16)
            n340 = Add(x=w563, y=w564) -> (x+y=w562:i16)
            n341 = call <vilib>:"NT Write Number.vi"("Numeric"=w562, "Name"=w561) -> ()  [unwired: 9 in, 1 out]
          }
          event "Test Ring": Value Change {
            # "When a test mode helper value is selected from the ring,\nset the tree item's variable to the string value"
            n342 = event-data() -> ("NewVal"=w571:u16)  [unwired: 1 in]
            n343 = property on="Test Ring" class="Ring (strict)"() -> ("Strings []"=w572:string[])  [unwired: 2 in, 2 out]
            n344 = Index Array(array=w572, index=w571) -> (element=w570:string)
            n345 = call <vilib>:"NT Write String.vi"("String"=w570, "Name"=w569) -> ()  [unwired: 9 in, 1 out]
          }
          event "Rec Mode": Value Change {
            # "Update globals for recording mode and path to read log from.\nClear when logging and let NetworkTables set path for vision to\nuse."
            n346 = event-data() -> ("NewVal"=w582:enum32{"Stop", "Record", "Playback"})  [unwired: 1 in]
            n347 = global write "WPI_DashboardLogging Global.vi" "Logging Filename"(path "") -> ()
            n348 = case shown="\"Playback\"" w582 {
              tunnel: w581 -> [_ w584 w592]
              tunnel: [_ _ w591] -> w578
              tunnel: [_ _ w590] -> _
              tunnel: w576 -> [_ _ w588]
              tunnel: cluster{i32, i32} {-250, 170} -> [_ _ w587]
              tunnel: [_ _ T38 {"Image Size"=TRUE, "Image Type"=TRUE, "Pixel Value"=TRUE, "ROI Information"=TRUE, "Zoom Factor"=FALSE} ("Image Information Shown:All Elements")] -> w574
              tunnel: [_ _ TRUE ("Zoom Factor")] -> w573
              frame Default {
              }
              frame "Stop", "Record" {
                # "Place Window too"
                n349 = invoke class="VI" method="FP.Close"(reference=w584) -> (reference out=w583:refnum<vi>)  [unwired: 2 in, 2 out]
                n350 = invoke class="VI" method="Abort VI"(reference=w583) -> ()  [unwired: 2 in, 3 out]
              }
              frame "Playback" {
                n351 = call "Open Playback Panel.vi"("Offset"=w587, "DB VI Ref"=w588, "Playback in"=w592) -> ("Playback out"=w589:refnum<vi>)  [unwired: 8 in]
                n352 = register-events(w589) -> (reference out=w591:refnum<event-registration>, error out=w590:errorcluster)  [unwired: 2 in]
              }
            }
            n353 = global write "WPI_DashboardLogging Global.vi" "Recording"(w582) -> ()
            n354 = property on="Camera Image" class="ImageControl"("Image Information Shown"=w574, "Image Information Visible"=w573) -> ()  [unwired: 2 in, 2 out]
            n355 = call <vilib>:"WPI_DashboardNT Log FieldName Cache.vi"("Operation"=enum16{"Lookup/Add", "Index", "Clear"}."Clear") -> ()  [unwired: 8 in, 3 out]
          }
          event Panel Close {
            w593 = enum32{"Stop", "Record", "Playback"}."Stop" ("Rec Mode")
            # "Playback window has been closed, abort"
            n356 = event-data() -> ()  [unwired: 1 in, 4 out]
            n357 = local write "Rec Mode"(w593) -> ()
            n358 = global write "WPI_DashboardLogging Global.vi" "Recording"(w593) -> ()
          }
          event Panel Close {
            # "Abort playback window and ourself"
            n359 = event-data() -> ()  [unwired: 1 in, 4 out]
            n360 = invoke class="VI" method="FP.Close"(reference=w598) -> (reference out=w597:refnum<vi>)  [unwired: 2 in, 2 out]
            n361 = invoke class="VI" method="Abort VI"(reference=w597) -> (error out=w596:errorcluster)  [unwired: 2 in, 2 out]
            n362 = invoke class="VI" method="Abort VI"(error in=w596) -> ()  [unwired: 2 in, 3 out]
          }
          event "Vision": Value Change {
            # "Enable/Disable Compression slider.\nHW USB is hard-coded into the camera"
            n363 = event-data() -> ("NewVal"=w604:u16)  [unwired: 1 in]
            n364 = Equal?(x=w604, y=u32 2 ("milliseconds to wait")) -> (x = y?=w602:bool)
            n365 = Select(t=T39."Disabled and Grayed Out" ("Disabled"), s=w602, f=T39."Enabled" ("Disabled")) -> (s? t:f=w599:T39)
            n366 = property on="Compression" class="Slide (strict)"("DisabledEnum"=w599) -> ()  [unwired: 2 in, 2 out]
          }
        }
      }
      n367 = property on="Camera Settings" class="Clust (strict)"("Val(Sgnl)"=w301) -> ()  [unwired: 2 in, 2 out]
      n368 = property on="On/Off" class="Bool (strict)"("Visible"=w300) -> ()  [unwired: 2 in, 2 out]
      n369 = property on="Motor" class="Clust (strict)"("Visible"=w300) -> ()  [unwired: 2 in, 2 out]
      n370 = property on="Progress" class="Clust (strict)"("Visible"=w300) -> ()  [unwired: 2 in, 2 out]
      n371 = property on="Test Ring" class="Ring (strict)"("Visible"=w300) -> ()  [unwired: 2 in, 2 out]
      n372 = property on="Rev/Fwd" class="Clust (strict)"("Visible"=w300) -> ()  [unwired: 2 in, 2 out]
      n373 = local write "DB Camera Config"(w300) -> ()
      n374 = property on="Camera Settings" class="Clust (strict)"("Visible"=w300) -> ()  [unwired: 2 in, 2 out]
      n375 = global write "WPI_DashboardLogging Global.vi" "Recording"(w304) -> ()
      n376 = local write "Rec Mode"(w304) -> ()
    }
    frame Enabled {
      # "More Unneeded Stuff (Hidden and Disabled)"
    }
  }
  n377 = while {
    stop <- FALSE stop-if-true
    # "Caption hover"
    n378 = Wait (ms)(milliseconds to wait=u32 100) -> ()  [unwired: 1 out]
    n379 = event shown="[7] \"Enable Notifications\": Mouse Enter" {
      selector: _ -> [_ _ _ _ _ _ _ _ _ _ _ _ _ _ _ _ _ _ _ _ _]
      dyn-events: _ -> [_ _ _ _ _ _ _ _ _ _ _ _ _ _ _ _ _ _ _ _ _]
      timeout: _ -> [_ _ _ _ _ _ _ _ _ _ _ _ _ _ _ _ _ _ _ _ _]
      tunnel: [TRUE _ _ _ _ _ _ _ _ _ _ _ _ _ _ _ _ _ _ _ _] -> w606
      event Timeout {
        n380 = event-data() -> ()  [unwired: 1 in, 3 out]
      }
      event "Clear PDP Sticky Faults": Mouse Enter {
        n381 = event-data() -> ()  [unwired: 1 in, 4 out]
        n382 = property on="Clear PDP Sticky Faults" class="Bool (strict)"("Caption.Visible"=TRUE) -> ()  [unwired: 2 in, 2 out]
      }
      event "Clear PDP Sticky Faults": Mouse Leave {
        n383 = event-data() -> ()  [unwired: 1 in, 4 out]
        n384 = property on="Clear PDP Sticky Faults" class="Bool (strict)"("Caption.Visible"=FALSE) -> ()  [unwired: 2 in, 2 out]
      }
      event "Reset Error Log": Mouse Enter {
        n385 = event-data() -> ()  [unwired: 1 in, 4 out]
        n386 = property on="Reset Error Log" class="Bool (strict)"("Caption.Visible"=TRUE) -> ()  [unwired: 2 in, 2 out]
      }
      event "Reset Error Log": Mouse Leave {
        n387 = event-data() -> ()  [unwired: 1 in, 4 out]
        n388 = property on="Reset Error Log" class="Bool (strict)"("Caption.Visible"=FALSE) -> ()  [unwired: 2 in, 2 out]
      }
      event "Reset PDP Energy": Mouse Enter {
        n389 = event-data() -> ()  [unwired: 1 in, 4 out]
        n390 = property on="Reset PDP Energy" class="Bool (strict)"("Caption.Visible"=TRUE) -> ()  [unwired: 2 in, 2 out]
      }
      event "Reset PDP Energy": Mouse Leave {
        n391 = event-data() -> ()  [unwired: 1 in, 4 out]
        n392 = property on="Reset PDP Energy" class="Bool (strict)"("Caption.Visible"=FALSE) -> ()  [unwired: 2 in, 2 out]
      }
      event "Enable Notifications": Mouse Enter {
        n393 = event-data() -> ()  [unwired: 1 in, 4 out]
        n394 = property on="Enable Notifications" class="Bool (strict)"("Caption.Visible"=TRUE) -> ()  [unwired: 2 in, 2 out]
      }
      event "Enable Notifications": Mouse Leave {
        n395 = event-data() -> ()  [unwired: 1 in, 4 out]
        n396 = property on="Enable Notifications" class="Bool (strict)"("Caption.Visible"=FALSE) -> ()  [unwired: 2 in, 2 out]
      }
      event "Dismiss Notification": Mouse Enter {
        n397 = event-data() -> ()  [unwired: 1 in, 4 out]
        n398 = property on="Dismiss Notification" class="Bool (strict)"("Caption.Visible"=TRUE) -> ()  [unwired: 2 in, 2 out]
      }
      event "Dismiss Notification": Mouse Leave {
        n399 = event-data() -> ()  [unwired: 1 in, 4 out]
        n400 = property on="Dismiss Notification" class="Bool (strict)"("Caption.Visible"=FALSE) -> ()  [unwired: 2 in, 2 out]
      }
      event "Clear Log": Mouse Enter {
        n401 = event-data() -> ()  [unwired: 1 in, 4 out]
        n402 = property on="Clear Log" class="Bool (strict)"("Caption.Visible"=TRUE) -> ()  [unwired: 2 in, 2 out]
      }
      event "Clear Log": Mouse Leave {
        n403 = event-data() -> ()  [unwired: 1 in, 4 out]
        n404 = property on="Clear Log" class="Bool (strict)"("Caption.Visible"=FALSE) -> ()  [unwired: 2 in, 2 out]
      }
      event "Top Left": Mouse Enter {
        n405 = event-data() -> ()  [unwired: 1 in, 4 out]
        n406 = property on="Top Left" class="Bool (strict)"("Caption.Visible"=TRUE) -> ()  [unwired: 2 in, 2 out]
      }
      event "Top Left": Mouse Leave {
        n407 = event-data() -> ()  [unwired: 1 in, 4 out]
        n408 = property on="Top Left" class="Bool (strict)"("Caption.Visible"=FALSE) -> ()  [unwired: 2 in, 2 out]
      }
      event "Top Right": Mouse Enter {
        n409 = event-data() -> ()  [unwired: 1 in, 4 out]
        n410 = property on="Top Right" class="Bool (strict)"("Caption.Visible"=TRUE) -> ()  [unwired: 2 in, 2 out]
      }
      event "Top Right": Mouse Leave {
        n411 = event-data() -> ()  [unwired: 1 in, 4 out]
        n412 = property on="Top Right" class="Bool (strict)"("Caption.Visible"=FALSE) -> ()  [unwired: 2 in, 2 out]
      }
      event "Bottom Left": Mouse Enter {
        n413 = event-data() -> ()  [unwired: 1 in, 4 out]
        n414 = property on="Bottom Left" class="Bool (strict)"("Caption.Visible"=TRUE) -> ()  [unwired: 2 in, 2 out]
      }
      event "Bottom Left": Mouse Leave {
        n415 = event-data() -> ()  [unwired: 1 in, 4 out]
        n416 = property on="Bottom Left" class="Bool (strict)"("Caption.Visible"=FALSE) -> ()  [unwired: 2 in, 2 out]
      }
      event "Bottom Right": Mouse Enter {
        n417 = event-data() -> ()  [unwired: 1 in, 4 out]
        n418 = property on="Bottom Right" class="Bool (strict)"("Caption.Visible"=TRUE) -> ()  [unwired: 2 in, 2 out]
      }
      event "Bottom Right": Mouse Leave {
        n419 = event-data() -> ()  [unwired: 1 in, 4 out]
        n420 = property on="Bottom Right" class="Bool (strict)"("Caption.Visible"=FALSE) -> ()  [unwired: 2 in, 2 out]
      }
    }
    n421 = property on="hover hint" class="Str"("Visible"=w606) -> ()  [unwired: 2 in, 2 out]
  }
  n422 = call "Initialize Camera and CheckList Mod.vi"() -> ("Cluster"=w4:cluster{"value":i32, "value":i32, "index":i32}, "Array"=w2:cluster{string[]}[], "File Refnum"=w3:T40)  [unwired: 9 in]
  n423 = while {
    shift-right: [w630] -> _
    shift-left: w3 -> [w631]
    tunnel: w2 -> [w632]
    stop <- FALSE stop-if-true
    n424 = event shown="[0] Timeout" {
      selector: _ -> [_ _ _ _]
      dyn-events: _ -> [_ _ _ _]
      timeout: 60 -> [_ _ _ _]
      tunnel: w632 -> [_ w636 w662 _]
      tunnel: w631 -> [w635 w638 w661 w673]
      tunnel: [w635 w637 w661 w673] -> w630
      event Timeout {
        n425 = event-data() -> ()  [unwired: 1 in, 3 out]
      }
      event "DB Camera Config": Value Change {
        # "Show or hide the cluster of controls, store in ini file"
        n426 = event-data() -> ("NewVal"=w639:bool)  [unwired: 1 in, 5 out]
        n427 = case shown="False" w639 {
          tunnel: w638 -> [w643 w660]
          tunnel: [w642 w660] -> w637
          tunnel: w636 -> [w641 _]
          frame False {
            w656 = "Camera"
            w645 = FALSE ("Visible")
            n428 = local read "Camera Settings"() -> (w644:T5)
            n429 = Index Array(array=w641) -> (element=w652:cluster{string[]})  [unwired: 1 in]
            n430 = Unbundle(w644) -> ("Frame Rate"=w649:i32, "Compression"=w648:i32, "Size"=w650:u16)
            n431 = Unbundle(w652) -> (w651:string[])
            n432 = Index Array(array=w651, index=w650) -> (element=w640:string)
            n433 = call-poly <vilib>:"Write Key.vi"("section"=w656, "value"=w640, "key"="Size", "refnum"=w643) -> ("refnum out"=w658:T40)  [unwired: 2 in, 5 out]
            n434 = call-poly <vilib>:"Write Key.vi"("section"=w656, "value"=w649, "key"="FrameRate", "refnum"=w658) -> ("refnum out"=w657:T40)  [unwired: 1 in, 6 out]
            n435 = local write "DB Camera Config"(w645) -> ()
            n436 = call-poly <vilib>:"Write Key.vi"("section"=w656, "value"=w648, "key"="Compression", "refnum"=w657) -> ("refnum out"=w646:T40)  [unwired: 1 in, 6 out]
            n437 = property on="Camera Settings" class="Clust (strict)"("Visible"=w645) -> ()  [unwired: 2 in, 2 out]
            n438 = call <vilib>:"Close Config Data.vi"("refnum"=w646) -> ("file path"=w647:path)  [unwired: 2 in, 8 out]
            n439 = call <vilib>:"Open Config Data.vi"("configuration file path"=w647) -> ("refnum"=w642:T40)  [unwired: 8 in, 2 out]
          }
          frame True {
            n440 = property on="Camera Settings" class="Clust (strict)"("Visible"=TRUE) -> ()  [unwired: 2 in, 2 out]
          }
        }
      }
      event "Camera Settings": Value Change {
        # "Update summary string when any elements of DB camera change"
        n441 = event-data() -> ("NewVal"=w663:T5)  [unwired: 1 in, 5 out]
        n442 = Index Array(array=w662) -> (element=w666:cluster{string[]})  [unwired: 1 in]
        n443 = Unbundle(w663) -> ("Frame Rate"=w670:i32, "Compression"=w671:i32, "Size"=w668:u16)
        n444 = Unbundle(w666) -> (w667:string[])
        n445 = Index Array(array=w667, index=w668) -> (element=w669:string)
        n446 = Format Into String(format string="%s   %dfps   %d%%", w669, w670, w671) -> (resulting string=w665:string)  [unwired: 2 in, 1 out]
        n447 = Build Array(w665) -> (w672:string[])
        n448 = property on="DB Camera Config" class="Bool (strict)"("Strings [4]"=w672) -> ()  [unwired: 2 in, 2 out]
      }
      event "Vision": Value Change {
        # "Enable/Disable Compression slider.\nHW USB is hard-coded into the camera"
        n449 = event-data() -> ("NewVal"=w675:u16)  [unwired: 1 in, 5 out]
        n450 = Equal?(x=w675, y=u32 2 ("milliseconds to wait")) -> (x = y?=w678:bool)
        n451 = Select(t=T39."Disabled and Grayed Out" ("Disabled"), s=w678, f=T39."Enabled" ("Disabled")) -> (s? t:f=w674:T39)
        n452 = property on="Compression" class="Slide (strict)"("DisabledEnum"=w674) -> ()  [unwired: 2 in, 2 out]
      }
    }
  }
  n453 = property on="Camera Settings" class="Clust (strict)"("Val(Sgnl)"=w4) -> ()  [unwired: 2 in, 2 out]
  n454 = property on="NotificationCluster" class="Clust (strict)"() -> ("Controls[]"=w14:refnum<vi>[])  [unwired: 2 in, 2 out]
  n455 = Index Array(array=w14) -> (element=w17:refnum<vi>)  [unwired: 1 in]
  n456 = To More Specific Class(target class=w16, reference=w17) -> (specific class reference=w18:refnum<vi>, error out=w12:errorcluster)  [unwired: 1 in]
  n457 = property class="MCListbox"(reference=w18, error in=w12, "SelColor"=u32 16723200 ("Round Color Box"), "NumCols"=u32 2 ("Number of Columns"), "ItemNames"=string[][] [] ("Item Names")) -> (reference out=w13:refnum<vi>, error out=w11:errorcluster)
  n458 = while {
    tunnel: w13 -> [w689]
    tunnel: w11 -> [w688]
    stop <- FALSE stop-if-true
    # "Log"
    # "Screen Location"
    # "Notifications"
    n459 = Wait (ms)(milliseconds to wait=u32 50) -> ()  [unwired: 1 out]
    n460 = property on="NotificationCluster" class="Clust (strict)"("Visible"="Notifications") -> ()  [unwired: 2 in, 2 out]
    n461 = local read "notification"() -> (w687:string)
    n462 = call "notification location.vi"("Bottom Right"="Bottom Right", "Bottom Left"="Bottom Left", "Top Right"="Top Right", "Top Left"="Top Left") -> ("ButtonStates"=w698:bool[], "Text Justification"=w699:enum16{"Left", "Center", "Right"}, "Position"=w700:T42)
    n463 = local read "Rail Voltages"() -> (w681:T15)
    n464 = Not(x="Enable Notifications") -> (.not. x?=w682:bool)
    n465 = Build Array (concatenate)(w698, w682) -> (w692:bool[])
    n466 = property on="notification" class="Str"("Position"=w700, "Text.Justify"=w699) -> ()  [unwired: 2 in, 2 out]
    n467 = call "notification log.vi"("Notification"=w687, "Clear Log"="Clear Log") -> ("Output Log"=w686:string[][])
    n468 = case shown="True" "Enable Notifications" {
      tunnel: [w738 w743] -> w708
      tunnel: [w738 w742] -> w707
      tunnel: "Dismiss Notification" -> [_ w741]
      tunnel: ["" ("Notification") w740] -> w706
      tunnel: w681 -> [_ w739]
      frame False {
        w738 = FALSE ("Blinking?")
      }
      frame True {
        n469 = call "fault notifications.vi"("Dismiss Notification"=w741, "Rail Voltages"=w739) -> ("Notification"=w740:string, "Blinking?"=w743:bool, "Visible?"=w742:bool)  [unwired: 11 in]
      }
    }
    "notification" <- w706
    n470 = call "Button_number.vi"("Button Array"=w692) -> ("Button Pressed"=w697:i32)
    n471 = case shown="True" "Enable Notifications" {
      tunnel: [T39."Disabled and Grayed Out" ("Disabled") T39."Enabled" ("Disabled")] -> w705
      frame False {
      }
      frame True {
      }
    }
    n472 = property class="MCListbox"(reference=w689, error in=w688, "ItemNames"=w686) -> ()  [unwired: 2 out]
    n473 = case shown="1" w697 {
      tunnel: [_ T39."Disabled and Grayed Out" ("Disabled") T39."Enabled" ("Disabled") T39."Enabled" ("Disabled") T39."Enabled" ("Disabled") T39."Disabled and Grayed Out" ("Disabled")] -> w696
      tunnel: [_ T39."Enabled" ("Disabled") T39."Disabled and Grayed Out" ("Disabled") T39."Enabled" ("Disabled") T39."Enabled" ("Disabled") T39."Disabled and Grayed Out" ("Disabled")] -> w695
      tunnel: [_ T39."Enabled" ("Disabled") T39."Enabled" ("Disabled") T39."Disabled and Grayed Out" ("Disabled") T39."Enabled" ("Disabled") T39."Disabled and Grayed Out" ("Disabled")] -> w694
      tunnel: [_ T39."Enabled" ("Disabled") T39."Enabled" ("Disabled") T39."Enabled" ("Disabled") T39."Disabled and Grayed Out" ("Disabled") T39."Disabled and Grayed Out" ("Disabled")] -> w693
      frame 0, Default {
      }
      frame 1 {
      }
      frame 2 {
      }
      frame 3 {
      }
      frame 4 {
      }
      frame 5 {
      }
    }
    n474 = case shown="False" w682 {
      tunnel: [T39."Enabled" ("Disabled") T39."Disabled and Grayed Out" ("Disabled")] -> w684
      tunnel: [T39."Enabled" ("Disabled") T39."Disabled and Grayed Out" ("Disabled")] -> w683
      frame False {
      }
      frame True {
      }
    }
    n475 = property on="Dismiss Notification" class="Bool (strict)"("DisabledEnum"=w705) -> ()  [unwired: 2 in, 2 out]
    n476 = property on="Clear Log" class="Bool (strict)"("DisabledEnum"=w684) -> ()  [unwired: 2 in, 2 out]
    n477 = property on="Notifications" class="Bool (strict)"("DisabledEnum"=w683) -> ()  [unwired: 2 in, 2 out]
    n478 = property on="notification" class="Str"("Blinking"=w708, "Visible"=w707) -> ()  [unwired: 2 in, 2 out]
    n479 = property on="Top Left" class="Bool (strict)"("DisabledEnum"=w696) -> ()  [unwired: 2 in, 2 out]
    n480 = property on="Top Right" class="Bool (strict)"("DisabledEnum"=w695) -> ()  [unwired: 2 in, 2 out]
    n481 = property on="Bottom Left" class="Bool (strict)"("DisabledEnum"=w694) -> ()  [unwired: 2 in, 2 out]
    n482 = property on="Bottom Right" class="Bool (strict)"("DisabledEnum"=w693) -> ()  [unwired: 2 in, 2 out]
    "Notifications" <- "Enable Notifications"
  }
